vi "torres hanoi.vi"() -> ()   [LabVIEW 2020]
uses:
  <vilib>/Utility/miscctls.llb/LVPoint32TypeDef.ctl
  <vilib>/Utility/miscctls.llb/LVPositionTypeDef.ctl
  <vilib>/Utility/miscctls.llb/LVBoundsTypeDef.ctl
panel:
  out "?":string
  out "solucion de inicio a final 5":string
  out "solucion de inicio a final 4":string
  in  "?":bool
  out "solucion de inicio a final 3":string
  out "result":bool
  out "Position 1":T1
  out "# de movimientos":dbl
  out "Position 2":T1
  out "Position 3":T1
  out "Position 4":T1
  out "Position 5":T1
  out "Position":T1
  in  "seleccione  # de discos:":u16(ring) items=["3"=3, "4"=4, "5"=5]
  out "Coords":T2
  in  "?":bool
  out "disco5":bool
  out "disco4":bool
  out "disco3":bool
  out "disco2":bool
  out "disco1":bool
  out "final":bool
  out "medio":bool
  out "inicio":bool
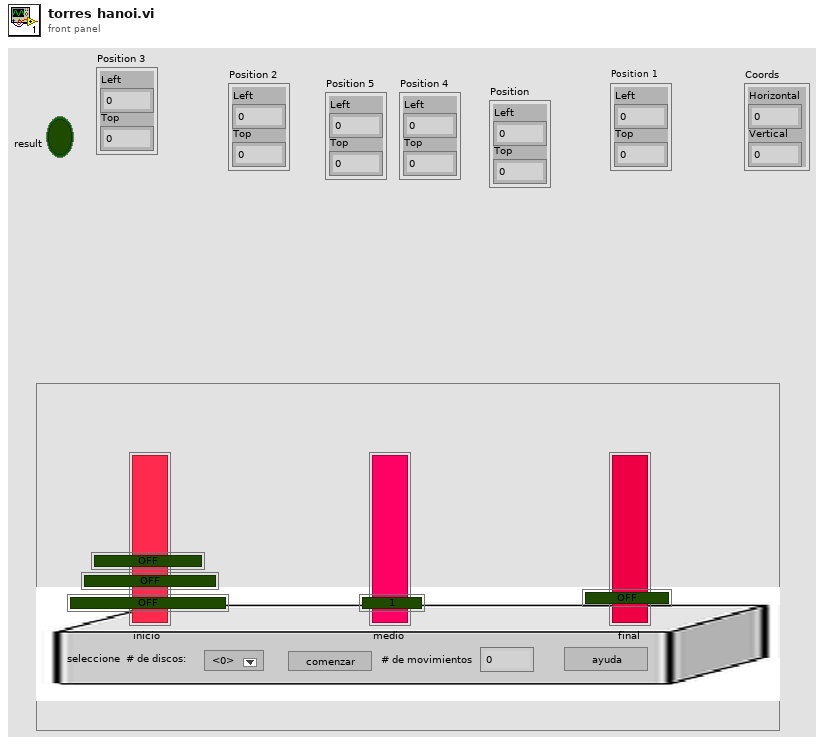
[diagram p1: front panel]
types:
  T1 = typedef "LVPositionTypeDef.ctl" = cluster{"Left":i32, "Top":i32}
  T2 = typedef "LVPoint32TypeDef.ctl" = cluster{"Horizontal":i32, "Vertical":i32}
  T3 = typedef "LVBoundsTypeDef.ctl" = cluster{"Width":u32, "Height":u32}
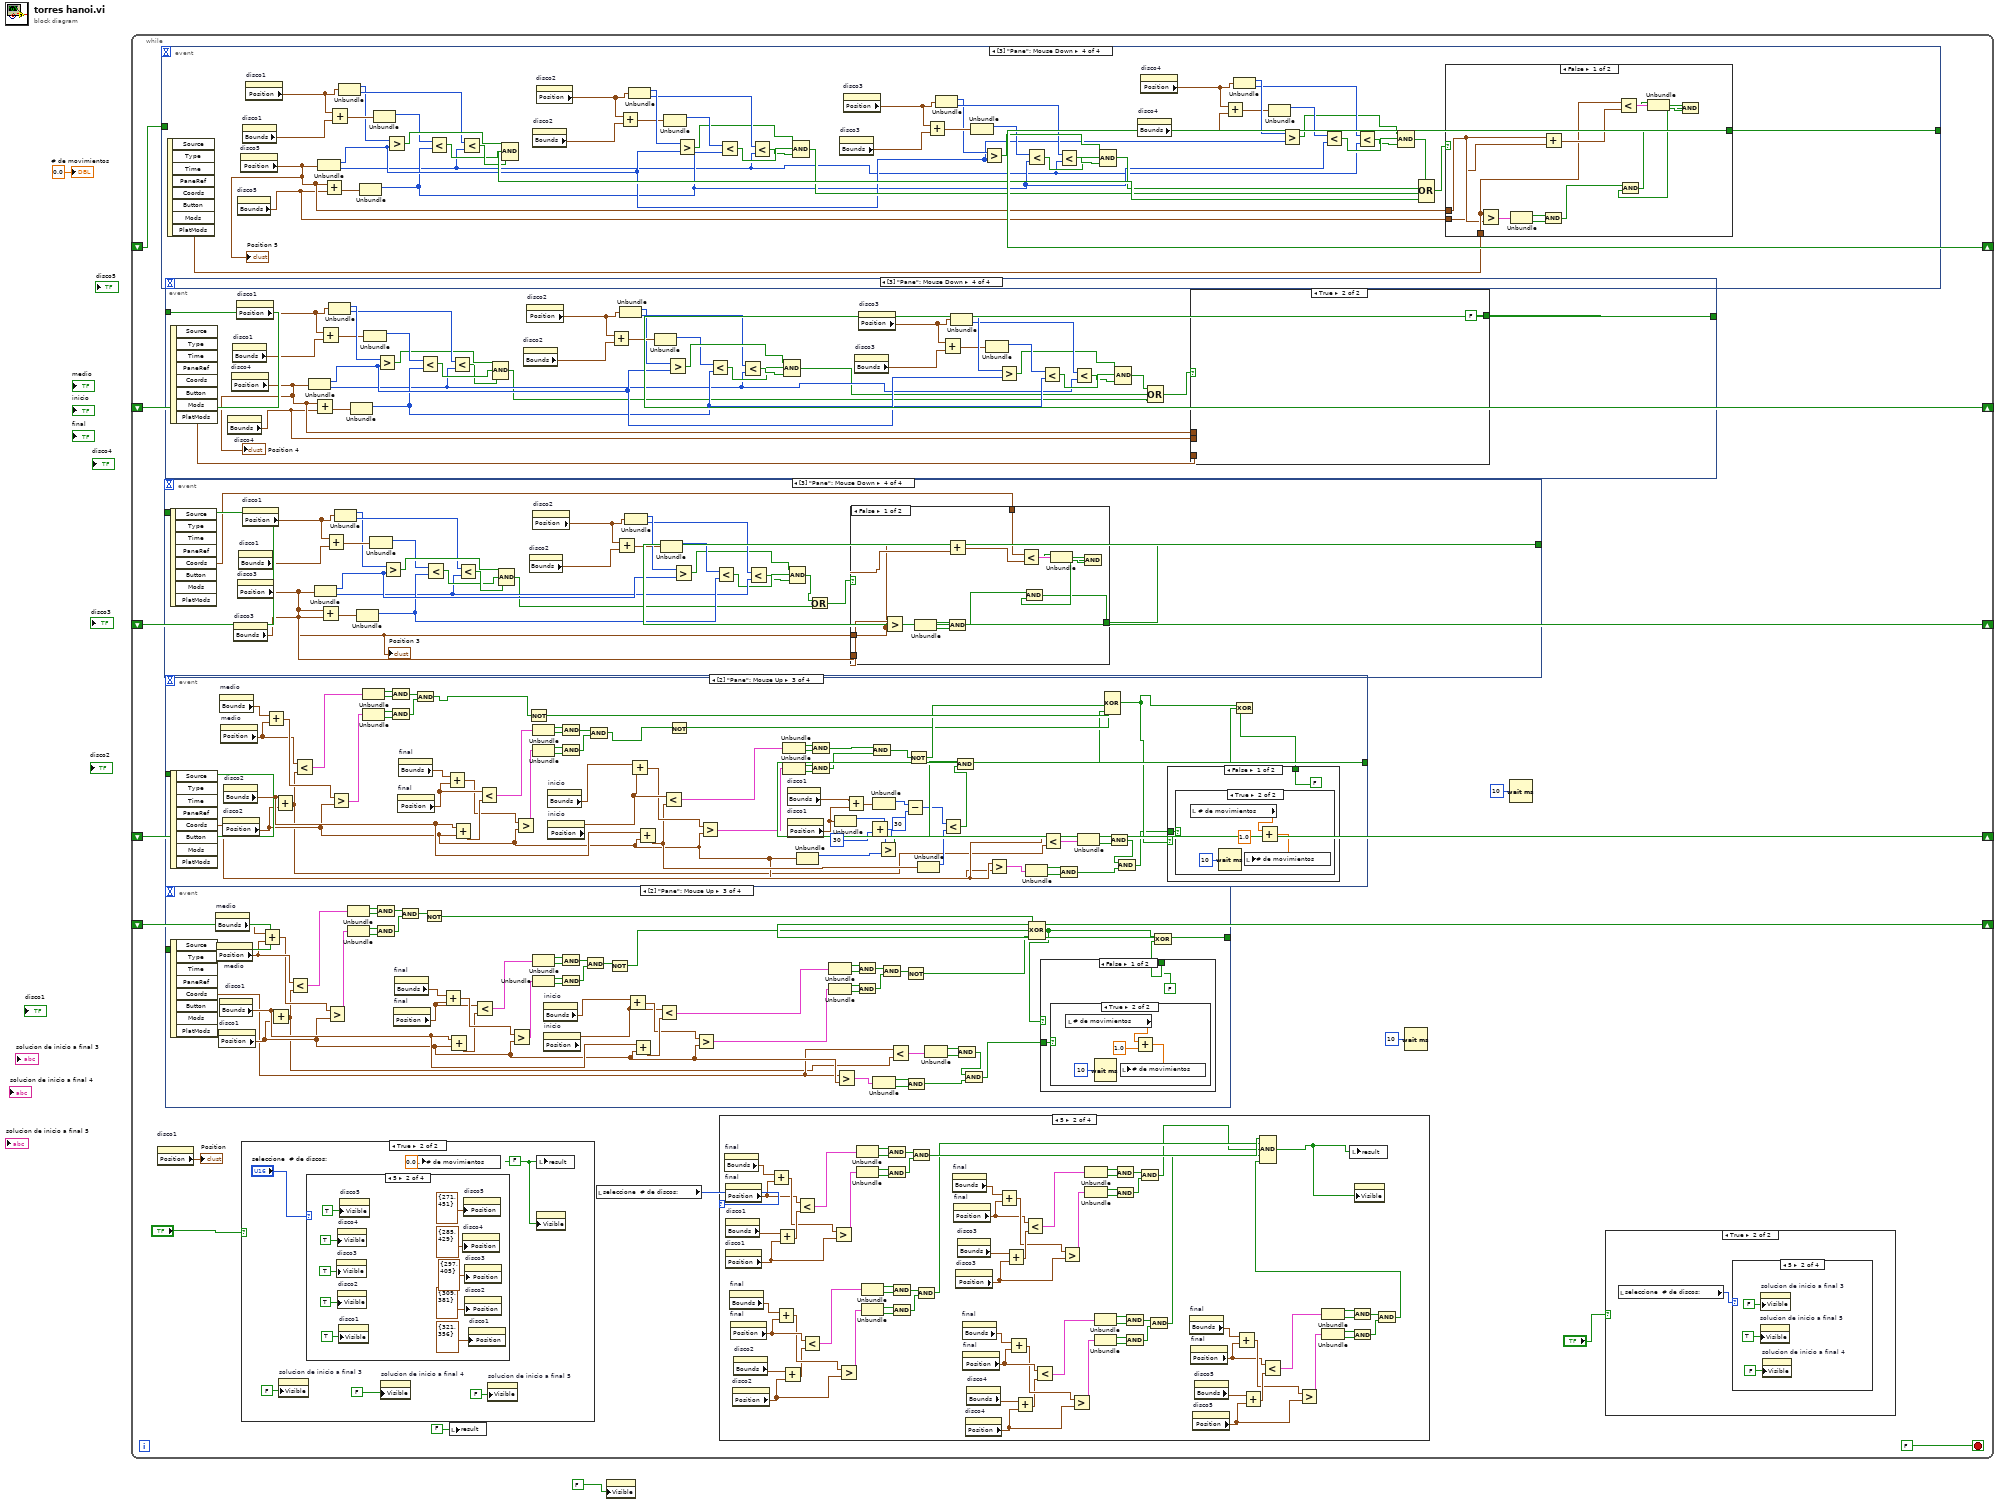
[diagram p0: block diagram]
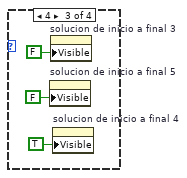
[diagram p4: hidden frame]
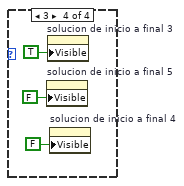
[diagram p5: hidden frame]
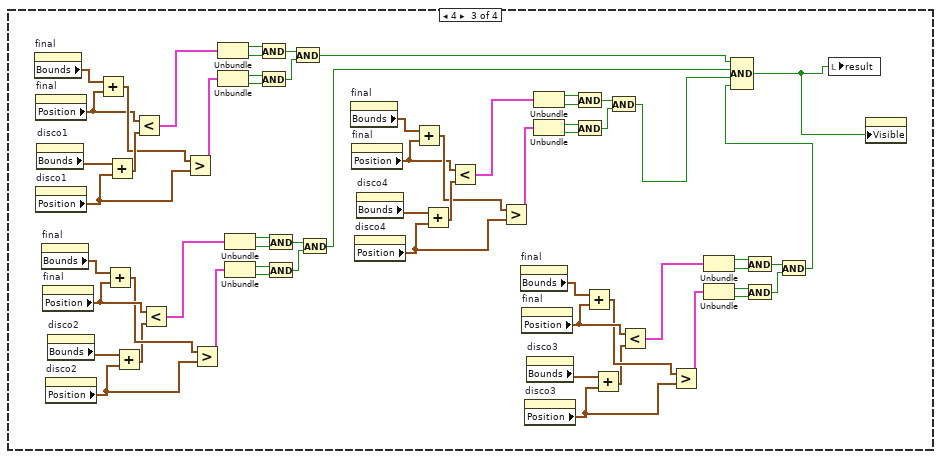
[diagram p7: hidden frame]
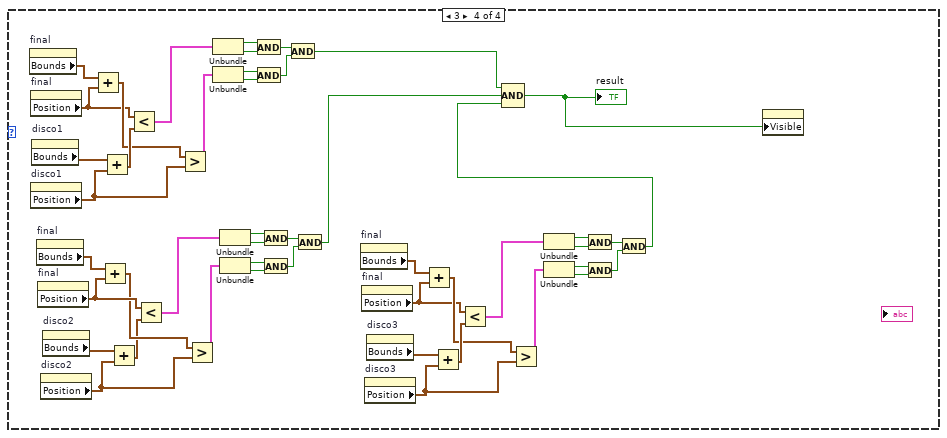
[diagram p8: hidden frame]
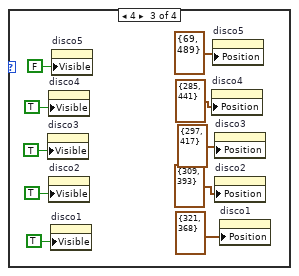
[diagram p11: hidden frame]
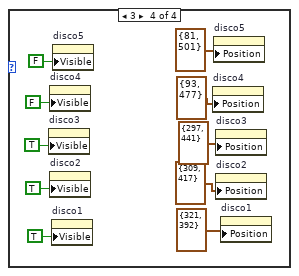
[diagram p12: hidden frame]
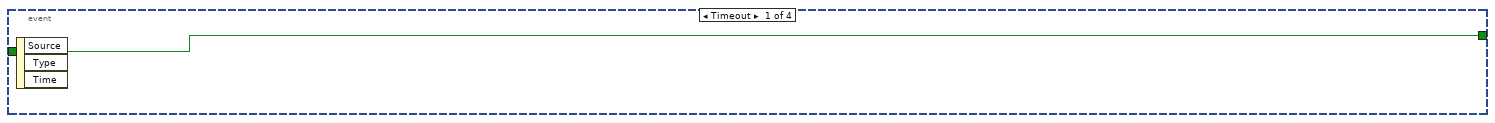
[diagram p13: hidden frame]
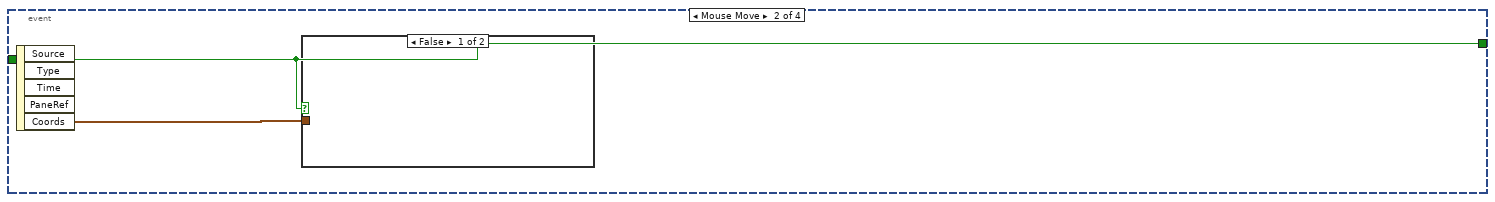
[diagram p14: hidden frame]
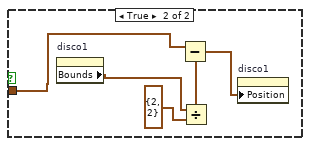
[diagram p15: hidden frame]
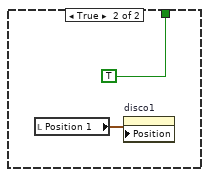
[diagram p17: hidden frame]
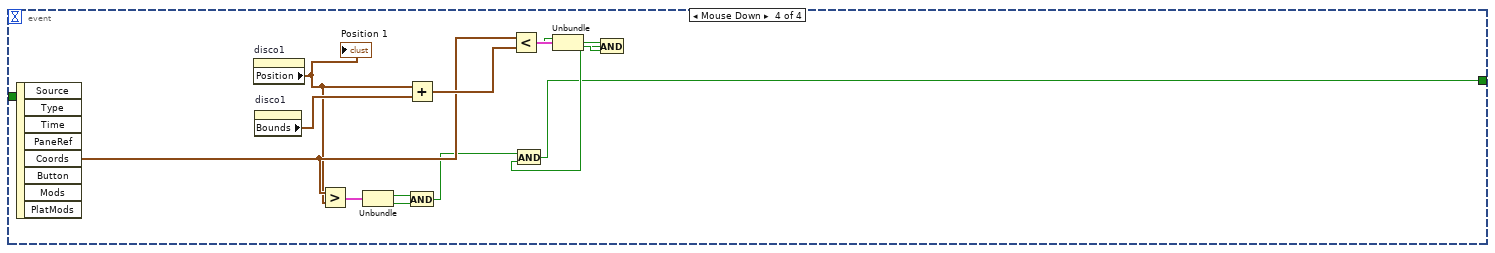
[diagram p18: hidden frame]
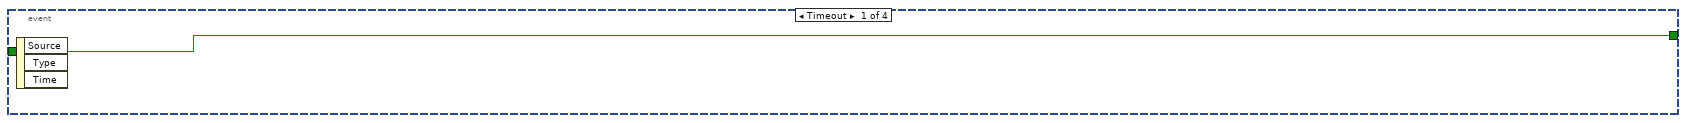
[diagram p19: hidden frame]
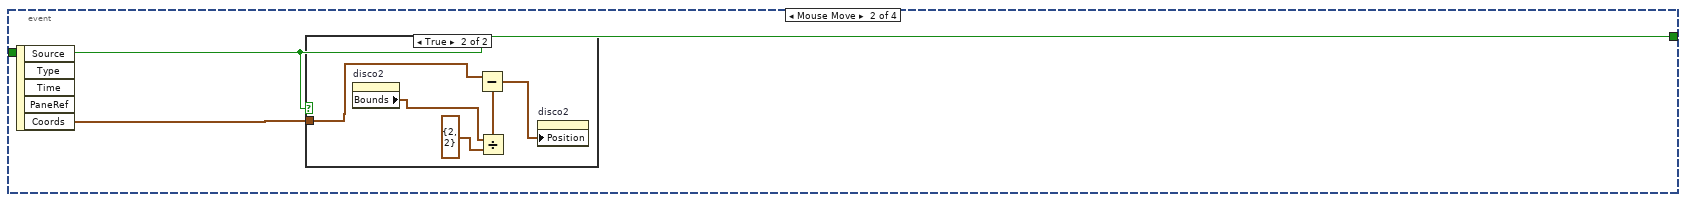
[diagram p20: hidden frame]
diagram:
  n1 = while {
    shift-right: [w18] -> _
    shift-left: _ -> [w19]
    shift-right: [w16] -> _
    shift-left: _ -> [w17]
    shift-right: [w14] -> _
    shift-left: _ -> [w15]
    shift-right: [w12] -> _
    shift-left: _ -> [w13]
    shift-right: [w10] -> _
    shift-left: _ -> [w11]
    stop <- FALSE stop-if-true
    n2 = property on="disco1" class="Bool (strict)"() -> ("Position"=→"Position":T1)  [unwired: 2 in, 2 out]
    n3 = event shown="[3] \"Pane\": Mouse Down" {
      selector: _ -> [_ _ _ _]
      dyn-events: _ -> [_ _ _ _]
      timeout: _ -> [_ _ _ _]
      tunnel: w19 -> [w764 w765 _ _]
      tunnel: [w764 w765 w836 w935] -> w18
      event Timeout {
        n4 = event-data() -> ()  [unwired: 1 in, 3 out]
      }
      event Mouse Move {
        n5 = event-data() -> ("Coords"=w766:T2)  [unwired: 1 in, 4 out]
        n6 = case shown="False" w765 {
          tunnel: w766 -> [_ w769]
          frame False {
          }
          frame True {
            n7 = property on="disco5" class="Bool (strict)"() -> ("Bounds"=w771:T3)  [unwired: 2 in, 2 out]
            n8 = Divide(x=w771, y=T3 {"Width"=2, "Height"=2}) -> (x/y=w768:cluster{"Width":dbl, "Height":dbl})
            n9 = Subtract(x=w769, y=w768) -> (x-y=w767:cluster{dbl, dbl})
            n10 = property on="disco5" class="Bool (strict)"("Position"=w767) -> ()  [unwired: 2 in, 2 out]
            "Coords" <- w769
          }
        }
      }
      event Mouse Up {
        n11 = event-data() -> ("Coords"=w774:T2)  [unwired: 1 in, 7 out]
        n12 = property on="medio" class="Bool (strict)"() -> ("Bounds"=w871:T3)  [unwired: 2 in, 2 out]
        n13 = property on="medio" class="Bool (strict)"() -> ("Position"=w870:T1)  [unwired: 2 in, 2 out]
        n14 = property on="disco5" class="Bool (strict)"() -> ("Position"=w773:T1)  [unwired: 2 in, 2 out]
        n15 = property on="disco5" class="Bool (strict)"() -> ("Bounds"=w842:T3)  [unwired: 2 in, 2 out]
        n16 = Add(x=w871, y=w870) -> (x+y=w869:T3)
        n17 = Add(x=w842, y=w773) -> (x+y=w772:T3)
        n18 = Less?(x=w870, y=w772) -> (x < y?=w873:cluster{bool, bool})
        n19 = Greater?(x=w869, y=w773) -> (0:w872:cluster{bool, bool})
        n20 = Unbundle(w873) -> (w877:bool, w876:bool)
        n21 = Unbundle(w872) -> (w879:bool, w878:bool)
        n22 = And(x=w877, y=w876) -> (x .and. y?=w874:bool)
        n23 = And(x=w879, y=w878) -> (x .and. y?=w875:bool)
        n24 = property on="final" class="Bool (strict)"() -> ("Position"=w855:T1)  [unwired: 2 in, 2 out]
        n25 = property on="final" class="Bool (strict)"() -> ("Bounds"=w856:T3)  [unwired: 2 in, 2 out]
        n26 = And(x=w874, y=w875) -> (x .and. y?=w868:bool)
        n27 = Not(x=w868) -> (.not. x?=w839:bool)
        n28 = Add(x=w856, y=w855) -> (x+y=w866:T3)
        n29 = Add(x=w842, y=w773) -> (x+y=w863:T3)
        n30 = Less?(x=w855, y=w863) -> (x < y?=w864:cluster{bool, bool})
        n31 = Greater?(x=w866, y=w773) -> (0:w865:cluster{bool, bool})
        n32 = Unbundle(w864) -> (w859:bool, w860:bool)
        n33 = Unbundle(w865) -> (w857:bool, w858:bool)
        n34 = property on="inicio" class="Bool (strict)"() -> ("Bounds"=w844:T3)  [unwired: 2 in, 2 out]
        n35 = property on="inicio" class="Bool (strict)"() -> ("Position"=w843:T1)  [unwired: 2 in, 2 out]
        n36 = And(x=w859, y=w860) -> (x .and. y?=w862:bool)
        n37 = And(x=w857, y=w858) -> (x .and. y?=w861:bool)
        n38 = And(x=w862, y=w861) -> (x .and. y?=w867:bool)
        n39 = Not(x=w867) -> (.not. x?=w840:bool)
        n40 = Add(x=w844, y=w843) -> (x+y=w846:T3)
        n41 = Add(x=w842, y=w773) -> (x+y=w824:T3)
        n42 = Less?(x=w843, y=w824) -> (x < y?=w848:cluster{bool, bool})
        n43 = Greater?(x=w846, y=w773) -> (0:w847:cluster{bool, bool})
        n44 = Unbundle(w848) -> (w852:bool, w851:bool)
        n45 = Unbundle(w847) -> (w854:bool, w853:bool)
        n46 = property on="disco1" class="Bool (strict)"() -> ("Bounds"=w830:T3)  [unwired: 2 in, 2 out]
        n47 = property on="disco1" class="Bool (strict)"() -> ("Position"=w831:T1)  [unwired: 2 in, 2 out]
        n48 = Unbundle(w773) -> ("Left"=w814:i32)  [unwired: 1 out]
        n49 = And(x=w852, y=w851) -> (x .and. y?=w849:bool)
        n50 = And(x=w854, y=w853) -> (x .and. y?=w850:bool)
        n51 = And(x=w849, y=w850) -> (x .and. y?=w845:bool)
        n52 = Unbundle(w831) -> ("Left"=w812:i32)  [unwired: 1 out]
        n53 = Add(x=w830, y=w831) -> (x+y=w832:T3)
        n54 = Not(x=w845) -> (.not. x?=w841:bool)
        n55 = Add(x=w812, y=30) -> (x+y=w810:i32)
        n56 = Greater?(x=w810, y=w814) -> (0:w826:bool)
        n57 = Unbundle(w832) -> ("Width"=w809:u32)  [unwired: 1 out]
        n58 = Subtract(x=w809, y=u32 30) -> (x-y=w807:u32)
        n59 = Unbundle(w824) -> ("Width"=w813:u32)  [unwired: 1 out]
        n60 = Less?(x=w807, y=w813) -> (x < y?=w825:bool)
        n61 = And(x=w826, y=w825) -> (x .and. y?=w784:bool)
        n62 = property on="disco2" class="Bool (strict)"() -> ("Bounds"=w829:T3)  [unwired: 2 in, 2 out]
        n63 = property on="disco2" class="Bool (strict)"() -> ("Position"=w828:T1)  [unwired: 2 in, 2 out]
        n64 = Unbundle(w828) -> ("Left"=w805:i32)  [unwired: 1 out]
        n65 = Add(x=w829, y=w828) -> (x+y=w827:T3)
        n66 = Add(x=w805, y=30) -> (x+y=w806:i32)
        n67 = Unbundle(w827) -> ("Width"=w803:u32)  [unwired: 1 out]
        n68 = Greater?(x=w806, y=w814) -> (0:w823:bool)
        n69 = Subtract(x=w803, y=u32 30) -> (x-y=w802:u32)
        n70 = Less?(x=w802, y=w813) -> (x < y?=w822:bool)
        n71 = And(x=w823, y=w822) -> (x .and. y?=w785:bool)
        n72 = property on="disco3" class="Bool (strict)"() -> ("Bounds"=w833:T3)  [unwired: 2 in, 2 out]
        n73 = property on="disco3" class="Bool (strict)"() -> ("Position"=w834:T1)  [unwired: 2 in, 2 out]
        n74 = Unbundle(w834) -> ("Left"=w800:i32)  [unwired: 1 out]
        n75 = Add(x=w833, y=w834) -> (x+y=w835:T3)
        n76 = Add(x=w800, y=30) -> (x+y=w799:i32)
        n77 = Unbundle(w835) -> ("Width"=w797:u32)  [unwired: 1 out]
        n78 = Greater?(x=w799, y=w814) -> (0:w821:bool)
        n79 = Subtract(x=w797, y=u32 30) -> (x-y=w796:u32)
        n80 = Less?(x=w796, y=w813) -> (x < y?=w820:bool)
        n81 = And(x=w821, y=w820) -> (x .and. y?=w786:bool)
        n82 = property on="disco4" class="Bool (strict)"() -> ("Bounds"=w817:T3)  [unwired: 2 in, 2 out]
        n83 = property on="disco4" class="Bool (strict)"() -> ("Position"=w816:T1)  [unwired: 2 in, 2 out]
        n84 = Unbundle(w816) -> ("Left"=w794:i32)  [unwired: 1 out]
        n85 = Add(x=w817, y=w816) -> (x+y=w815:T3)
        n86 = Add(x=w794, y=30) -> (x+y=w793:i32)
        n87 = Greater?(x=w793, y=w814) -> (0:w818:bool)
        n88 = Unbundle(w815) -> ("Width"=w791:u32)  [unwired: 1 out]
        n89 = Subtract(x=w791, y=u32 30) -> (x-y=w789:u32)
        n90 = Less?(x=w789, y=w813) -> (x < y?=w819:bool)
        n91 = And(x=w818, y=w819) -> (x .and. y?=w787:bool)
        n92 = Compound Arithmetic op=OR(w784, w785, w786, w787) -> (w788:bool)
        n93 = Greater?(x=w774, y=w773) -> (0:w783:cluster{bool, bool})
        n94 = Unbundle(w783) -> (w781:bool, w780:bool)
        n95 = Less?(x=w774, y=w772) -> (x < y?=w782:cluster{bool, bool})
        n96 = And(x=w781, y=w780) -> (x .and. y?=w776:bool)
        n97 = Unbundle(w782) -> (w779:bool, w778:bool)
        n98 = And(x=w779, y=w778) -> (x .and. y?=w777:bool)
        n99 = And(x=w777, y=w776) -> (x .and. y?=w775:bool)
        n100 = Compound Arithmetic op=XOR(w839, w840, w841, w788) -> (w837:bool)
        n101 = case shown="False" w837 {
          tunnel: [FALSE ("Accepted?") TRUE ("Accepted?")] -> w838
          tunnel: w775 -> [w880 _]
          frame False {
            n102 = case shown="True" w880 {
              frame False {
              }
              frame True {
                n103 = local read "# de movimientos"() -> (w884:dbl)
                n104 = Wait (ms)(milliseconds to wait=u32 10) -> ()  [unwired: 1 out]
                n105 = Add(x=w884, y=1.0) -> (x+y=w885:dbl)
                n106 = local write "# de movimientos"(w885) -> ()
              }
            }
          }
          frame True {
            n107 = local read "Position 5"() -> (w887:T1)
            n108 = property on="disco5" class="Bool (strict)"("Position"=w887) -> ()  [unwired: 2 in, 2 out]
          }
        }
        n109 = Exclusive Or(1:w838, 2:w837) -> (0:w836:bool)
      }
      event Mouse Down {
        n110 = event-data() -> ("Coords"=w936:T2)  [unwired: 1 in, 7 out]
        n111 = property on="disco5" class="Bool (strict)"() -> ("Bounds"=w902:T3)  [unwired: 2 in, 2 out]
        n112 = property on="disco5" class="Bool (strict)"() -> ("Position"=w903:T1)  [unwired: 2 in, 2 out]
        "Position 5" <- w903
        n113 = property on="disco1" class="Bool (strict)"() -> ("Bounds"=w913:T3)  [unwired: 2 in, 2 out]
        n114 = property on="disco1" class="Bool (strict)"() -> ("Position"=w914:T1)  [unwired: 2 in, 2 out]
        n115 = Unbundle(w903) -> ("Left"=w891:i32, "Top"=w889:i32)
        n116 = Add(x=w903, y=w902) -> (x+y=w917:T3)
        n117 = Add(x=w914, y=w913) -> (x+y=w916:T3)
        n118 = Unbundle(w914) -> ("Left"=w915:i32, "Top"=w919:i32)
        n119 = Unbundle(w917) -> ("Width"=w890:u32)  [unwired: 1 out]
        n120 = Unbundle(w916) -> ("Width"=w918:u32)  [unwired: 1 out]
        n121 = Greater?(x=w915, y=w891) -> (0:w920:bool)
        n122 = Less?(x=w918, y=w890) -> (x < y?=w921:bool)
        n123 = Less?(x=w919, y=w889) -> (x < y?=w922:bool)
        n124 = Compound Arithmetic op=AND(w920, w921, w922) -> (w934:bool)
        n125 = property on="disco2" class="Bool (strict)"() -> ("Bounds"=w912:T3)  [unwired: 2 in, 2 out]
        n126 = property on="disco2" class="Bool (strict)"() -> ("Position"=w911:T1)  [unwired: 2 in, 2 out]
        n127 = Add(x=w911, y=w912) -> (x+y=w909:T3)
        n128 = Unbundle(w911) -> ("Left"=w910:i32, "Top"=w907:i32)
        n129 = Unbundle(w909) -> ("Width"=w908:u32)  [unwired: 1 out]
        n130 = Greater?(x=w910, y=w891) -> (0:w906:bool)
        n131 = Less?(x=w908, y=w890) -> (x < y?=w905:bool)
        n132 = Less?(x=w907, y=w889) -> (x < y?=w904:bool)
        n133 = Compound Arithmetic op=AND(w906, w905, w904) -> (w933:bool)
        n134 = property on="disco3" class="Bool (strict)"() -> ("Bounds"=w923:T3)  [unwired: 2 in, 2 out]
        n135 = property on="disco3" class="Bool (strict)"() -> ("Position"=w924:T1)  [unwired: 2 in, 2 out]
        n136 = Add(x=w924, y=w923) -> (x+y=w926:T3)
        n137 = Unbundle(w924) -> ("Left"=w925:i32, "Top"=w928:i32)
        n138 = Unbundle(w926) -> ("Width"=w927:u32)  [unwired: 1 out]
        n139 = Greater?(x=w925, y=w891) -> (0:w929:bool)
        n140 = Less?(x=w927, y=w890) -> (x < y?=w930:bool)
        n141 = Less?(x=w928, y=w889) -> (x < y?=w931:bool)
        n142 = Compound Arithmetic op=AND(w929, w930, w931) -> (w932:bool)
        n143 = property on="disco4" class="Bool (strict)"() -> ("Bounds"=w901:T3)  [unwired: 2 in, 2 out]
        n144 = property on="disco4" class="Bool (strict)"() -> ("Position"=w900:T1)  [unwired: 2 in, 2 out]
        n145 = Add(x=w900, y=w901) -> (x+y=w898:T3)
        n146 = Unbundle(w900) -> ("Left"=w899:i32, "Top"=w896:i32)
        n147 = Unbundle(w898) -> ("Width"=w897:u32)  [unwired: 1 out]
        n148 = Greater?(x=w899, y=w891) -> (0:w895:bool)
        n149 = Less?(x=w897, y=w890) -> (x < y?=w894:bool)
        n150 = Less?(x=w896, y=w889) -> (x < y?=w893:bool)
        n151 = Compound Arithmetic op=AND(w895, w894, w893) -> (w892:bool)
        n152 = Compound Arithmetic op=OR(w892, w932, w933, w934) -> (w888:bool)
        n153 = case shown="False" w888 {
          tunnel: w936 -> [w948 _]
          tunnel: [w939 FALSE] -> w935
          tunnel: w903 -> [w938 _]
          tunnel: w902 -> [w937 _]
          frame False {
            n154 = Greater?(x=w948, y=w938) -> (0:w947:cluster{bool, bool})
            n155 = Unbundle(w947) -> (w943:bool, w942:bool)
            n156 = Add(x=w938, y=w937) -> (x+y=w949:T3)
            n157 = And(x=w943, y=w942) -> (x .and. y?=w940:bool)
            n158 = Less?(x=w948, y=w949) -> (x < y?=w946:cluster{bool, bool})
            n159 = Unbundle(w946) -> (w945:bool, w944:bool)
            n160 = And(x=w945, y=w944) -> (x .and. y?=w941:bool)
            n161 = And(x=w940, y=w941) -> (x .and. y?=w939:bool)
          }
          frame True {
          }
        }
      }
    }
    n162 = event shown="[3] \"Pane\": Mouse Down" {
      selector: _ -> [_ _ _ _]
      dyn-events: _ -> [_ _ _ _]
      timeout: _ -> [_ _ _ _]
      tunnel: w15 -> [w456 w457 _ _]
      tunnel: [w456 w457 w504 w583] -> w14
      event Timeout {
        n163 = event-data() -> ()  [unwired: 1 in, 3 out]
      }
      event Mouse Move {
        n164 = event-data() -> ("Coords"=w458:T2)  [unwired: 1 in, 4 out]
        n165 = case shown="False" w457 {
          tunnel: w458 -> [_ w462]
          frame False {
          }
          frame True {
            n166 = property on="disco3" class="Bool (strict)"() -> ("Bounds"=w460:T3)  [unwired: 2 in, 2 out]
            n167 = Divide(x=w460, y=T3 {"Width"=2, "Height"=2}) -> (x/y=w461:cluster{"Width":dbl, "Height":dbl})
            n168 = Subtract(x=w462, y=w461) -> (x-y=w459:cluster{dbl, dbl})
            n169 = property on="disco3" class="Bool (strict)"("Position"=w459) -> ()  [unwired: 2 in, 2 out]
          }
        }
      }
      event Mouse Up {
        n170 = event-data() -> ("Coords"=w466:T2)  [unwired: 1 in, 7 out]
        n171 = property on="medio" class="Bool (strict)"() -> ("Bounds"=w539:T3)  [unwired: 2 in, 2 out]
        n172 = property on="medio" class="Bool (strict)"() -> ("Position"=w538:T1)  [unwired: 2 in, 2 out]
        n173 = property on="disco3" class="Bool (strict)"() -> ("Position"=w465:T1)  [unwired: 2 in, 2 out]
        n174 = property on="disco3" class="Bool (strict)"() -> ("Bounds"=w510:T3)  [unwired: 2 in, 2 out]
        n175 = Add(x=w539, y=w538) -> (x+y=w537:T3)
        n176 = Add(x=w510, y=w465) -> (x+y=w464:T3)
        n177 = Less?(x=w538, y=w464) -> (x < y?=w541:cluster{bool, bool})
        n178 = Greater?(x=w537, y=w465) -> (0:w540:cluster{bool, bool})
        n179 = Unbundle(w541) -> (w545:bool, w544:bool)
        n180 = Unbundle(w540) -> (w547:bool, w546:bool)
        n181 = And(x=w545, y=w544) -> (x .and. y?=w542:bool)
        n182 = And(x=w547, y=w546) -> (x .and. y?=w543:bool)
        n183 = property on="final" class="Bool (strict)"() -> ("Position"=w523:T1)  [unwired: 2 in, 2 out]
        n184 = property on="final" class="Bool (strict)"() -> ("Bounds"=w524:T3)  [unwired: 2 in, 2 out]
        n185 = And(x=w542, y=w543) -> (x .and. y?=w536:bool)
        n186 = Not(x=w536) -> (.not. x?=w507:bool)
        n187 = Add(x=w524, y=w523) -> (x+y=w534:T3)
        n188 = Add(x=w510, y=w465) -> (x+y=w531:T3)
        n189 = Less?(x=w523, y=w531) -> (x < y?=w532:cluster{bool, bool})
        n190 = Greater?(x=w534, y=w465) -> (0:w533:cluster{bool, bool})
        n191 = Unbundle(w532) -> (w527:bool, w528:bool)
        n192 = Unbundle(w533) -> (w525:bool, w526:bool)
        n193 = property on="inicio" class="Bool (strict)"() -> ("Bounds"=w512:T3)  [unwired: 2 in, 2 out]
        n194 = property on="inicio" class="Bool (strict)"() -> ("Position"=w511:T1)  [unwired: 2 in, 2 out]
        n195 = And(x=w527, y=w528) -> (x .and. y?=w530:bool)
        n196 = And(x=w525, y=w526) -> (x .and. y?=w529:bool)
        n197 = And(x=w530, y=w529) -> (x .and. y?=w535:bool)
        n198 = Not(x=w535) -> (.not. x?=w508:bool)
        n199 = Add(x=w512, y=w511) -> (x+y=w514:T3)
        n200 = Add(x=w510, y=w465) -> (x+y=w500:T3)
        n201 = Less?(x=w511, y=w500) -> (x < y?=w516:cluster{bool, bool})
        n202 = Greater?(x=w514, y=w465) -> (0:w515:cluster{bool, bool})
        n203 = Unbundle(w516) -> (w520:bool, w519:bool)
        n204 = Unbundle(w515) -> (w522:bool, w521:bool)
        n205 = And(x=w520, y=w519) -> (x .and. y?=w517:bool)
        n206 = And(x=w522, y=w521) -> (x .and. y?=w518:bool)
        n207 = And(x=w517, y=w518) -> (x .and. y?=w513:bool)
        n208 = property on="disco1" class="Bool (strict)"() -> ("Bounds"=w501:T3)  [unwired: 2 in, 2 out]
        n209 = property on="disco1" class="Bool (strict)"() -> ("Position"=w502:T1)  [unwired: 2 in, 2 out]
        n210 = Unbundle(w465) -> ("Left"=w494:i32)  [unwired: 1 out]
        n211 = Not(x=w513) -> (.not. x?=w509:bool)
        n212 = Unbundle(w502) -> ("Left"=w490:i32)  [unwired: 1 out]
        n213 = Add(x=w501, y=w502) -> (x+y=w503:T3)
        n214 = Add(x=w490, y=30) -> (x+y=w489:i32)
        n215 = Unbundle(w503) -> ("Width"=w486:u32)  [unwired: 1 out]
        n216 = Greater?(x=w489, y=w494) -> (0:w499:bool)
        n217 = Subtract(x=w486, y=u32 30) -> (x-y=w487:u32)
        n218 = Unbundle(w500) -> ("Width"=w493:u32)  [unwired: 1 out]
        n219 = Less?(x=w487, y=w493) -> (x < y?=w498:bool)
        n220 = And(x=w499, y=w498) -> (x .and. y?=w477:bool)
        n221 = property on="disco2" class="Bool (strict)"() -> ("Bounds"=w497:T3)  [unwired: 2 in, 2 out]
        n222 = property on="disco2" class="Bool (strict)"() -> ("Position"=w496:T1)  [unwired: 2 in, 2 out]
        n223 = Unbundle(w496) -> ("Left"=w484:i32)  [unwired: 1 out]
        n224 = Add(x=w497, y=w496) -> (x+y=w495:T3)
        n225 = Add(x=w484, y=30) -> (x+y=w483:i32)
        n226 = Unbundle(w495) -> ("Width"=w481:u32)  [unwired: 1 out]
        n227 = Greater?(x=w483, y=w494) -> (0:w491:bool)
        n228 = Subtract(x=w481, y=u32 30) -> (x-y=w480:u32)
        n229 = Less?(x=w480, y=w493) -> (x < y?=w492:bool)
        n230 = And(x=w491, y=w492) -> (x .and. y?=w478:bool)
        n231 = Or(x=w477, y=w478) -> (x .or. y?=w476:bool)
        n232 = Greater?(x=w466, y=w465) -> (0:w475:cluster{bool, bool})
        n233 = Unbundle(w475) -> (w473:bool, w472:bool)
        n234 = Less?(x=w466, y=w464) -> (x < y?=w474:cluster{bool, bool})
        n235 = And(x=w473, y=w472) -> (x .and. y?=w468:bool)
        n236 = Unbundle(w474) -> (w471:bool, w470:bool)
        n237 = And(x=w471, y=w470) -> (x .and. y?=w469:bool)
        n238 = And(x=w469, y=w468) -> (x .and. y?=w467:bool)
        n239 = Compound Arithmetic op=XOR(w507, w508, w509, w476) -> (w505:bool)
        n240 = case shown="False" w505 {
          tunnel: [FALSE ("Accepted?") TRUE ("Accepted?")] -> w506
          tunnel: w467 -> [w548 _]
          frame False {
            n241 = case shown="True" w548 {
              frame False {
              }
              frame True {
                n242 = local read "# de movimientos"() -> (w552:dbl)
                n243 = Wait (ms)(milliseconds to wait=u32 10) -> ()  [unwired: 1 out]
                n244 = Add(x=w552, y=1.0) -> (x+y=w553:dbl)
                n245 = local write "# de movimientos"(w553) -> ()
              }
            }
          }
          frame True {
            n246 = local read "Position 3"() -> (w555:T1)
            n247 = property on="disco3" class="Bool (strict)"("Position"=w555) -> ()  [unwired: 2 in, 2 out]
          }
        }
        n248 = Exclusive Or(1:w506, 2:w505) -> (0:w504:bool)
      }
      event Mouse Down {
        n249 = event-data() -> ("Coords"=w584:T2)  [unwired: 1 in, 7 out]
        n250 = property on="disco3" class="Bool (strict)"() -> ("Bounds"=w572:T3)  [unwired: 2 in, 2 out]
        n251 = property on="disco3" class="Bool (strict)"() -> ("Position"=w571:T1)  [unwired: 2 in, 2 out]
        "Position 3" <- w571
        n252 = property on="disco1" class="Bool (strict)"() -> ("Bounds"=w573:T3)  [unwired: 2 in, 2 out]
        n253 = property on="disco1" class="Bool (strict)"() -> ("Position"=w574:T1)  [unwired: 2 in, 2 out]
        n254 = Unbundle(w571) -> ("Left"=w563:i32, "Top"=w561:i32)
        n255 = Add(x=w571, y=w572) -> (x+y=w577:T3)
        n256 = Add(x=w574, y=w573) -> (x+y=w576:T3)
        n257 = Unbundle(w574) -> ("Left"=w575:i32, "Top"=w579:i32)
        n258 = Unbundle(w577) -> ("Width"=w562:u32)  [unwired: 1 out]
        n259 = Unbundle(w576) -> ("Width"=w578:u32)  [unwired: 1 out]
        n260 = Greater?(x=w575, y=w563) -> (0:w580:bool)
        n261 = Less?(x=w578, y=w562) -> (x < y?=w581:bool)
        n262 = Less?(x=w579, y=w561) -> (x < y?=w582:bool)
        n263 = Compound Arithmetic op=AND(w580, w581, w582) -> (w556:bool)
        n264 = property on="disco2" class="Bool (strict)"() -> ("Bounds"=w570:T3)  [unwired: 2 in, 2 out]
        n265 = property on="disco2" class="Bool (strict)"() -> ("Position"=w569:T1)  [unwired: 2 in, 2 out]
        n266 = Add(x=w569, y=w570) -> (x+y=w567:T3)
        n267 = Unbundle(w569) -> ("Left"=w568:i32, "Top"=w565:i32)
        n268 = Unbundle(w567) -> ("Width"=w566:u32)  [unwired: 1 out]
        n269 = Greater?(x=w568, y=w563) -> (0:w564:bool)
        n270 = Less?(x=w566, y=w562) -> (x < y?=w560:bool)
        n271 = Less?(x=w565, y=w561) -> (x < y?=w559:bool)
        n272 = Compound Arithmetic op=AND(w564, w560, w559) -> (w557:bool)
        n273 = Or(x=w557, y=w556) -> (x .or. y?=w558:bool)
        n274 = case shown="False" w558 {
          tunnel: w584 -> [w588 _]
          tunnel: [w587 FALSE] -> w583
          tunnel: w572 -> [w586 _]
          tunnel: w571 -> [w585 _]
          frame False {
            n275 = Greater?(x=w588, y=w585) -> (0:w596:cluster{bool, bool})
            n276 = Unbundle(w596) -> (w592:bool, w591:bool)
            n277 = Add(x=w585, y=w586) -> (x+y=w597:T3)
            n278 = And(x=w592, y=w591) -> (x .and. y?=w589:bool)
            n279 = Less?(x=w588, y=w597) -> (x < y?=w595:cluster{bool, bool})
            n280 = Unbundle(w595) -> (w594:bool, w593:bool)
            n281 = And(x=w594, y=w593) -> (x .and. y?=w590:bool)
            n282 = And(x=w589, y=w590) -> (x .and. y?=w587:bool)
          }
          frame True {
          }
        }
      }
    }
    n283 = event shown="[3] \"Pane\": Mouse Down" {
      selector: _ -> [_ _ _ _]
      dyn-events: _ -> [_ _ _ _]
      timeout: _ -> [_ _ _ _]
      tunnel: w17 -> [w599 w600 _ _]
      tunnel: [w599 w600 w660 w748] -> w16
      event Timeout {
        n284 = event-data() -> ()  [unwired: 1 in, 3 out]
      }
      event Mouse Move {
        n285 = event-data() -> ("Coords"=w601:T2)  [unwired: 1 in, 4 out]
        n286 = case shown="False" w600 {
          tunnel: w601 -> [_ w602]
          frame False {
          }
          frame True {
            n287 = property on="disco4" class="Bool (strict)"() -> ("Bounds"=w604:T3)  [unwired: 2 in, 2 out]
            n288 = Divide(x=w604, y=T3 {"Width"=2, "Height"=2}) -> (x/y=w605:cluster{"Width":dbl, "Height":dbl})
            n289 = Subtract(x=w602, y=w605) -> (x-y=w603:cluster{dbl, dbl})
            n290 = property on="disco4" class="Bool (strict)"("Position"=w603) -> ()  [unwired: 2 in, 2 out]
          }
        }
      }
      event Mouse Up {
        n291 = event-data() -> ("Coords"=w609:T2)  [unwired: 1 in, 7 out]
        n292 = property on="medio" class="Bool (strict)"() -> ("Bounds"=w669:T3)  [unwired: 2 in, 2 out]
        n293 = property on="medio" class="Bool (strict)"() -> ("Position"=w670:T1)  [unwired: 2 in, 2 out]
        n294 = property on="disco4" class="Bool (strict)"() -> ("Position"=w608:T1)  [unwired: 2 in, 2 out]
        n295 = property on="disco4" class="Bool (strict)"() -> ("Bounds"=w698:T3)  [unwired: 2 in, 2 out]
        n296 = Add(x=w669, y=w670) -> (x+y=w671:T3)
        n297 = Add(x=w698, y=w608) -> (x+y=w607:T3)
        n298 = Less?(x=w670, y=w607) -> (x < y?=w667:cluster{bool, bool})
        n299 = Greater?(x=w671, y=w608) -> (0:w668:cluster{bool, bool})
        n300 = Unbundle(w667) -> (w663:bool, w664:bool)
        n301 = Unbundle(w668) -> (w661:bool, w662:bool)
        n302 = And(x=w663, y=w664) -> (x .and. y?=w666:bool)
        n303 = And(x=w661, y=w662) -> (x .and. y?=w665:bool)
        n304 = property on="final" class="Bool (strict)"() -> ("Position"=w685:T1)  [unwired: 2 in, 2 out]
        n305 = property on="final" class="Bool (strict)"() -> ("Bounds"=w684:T3)  [unwired: 2 in, 2 out]
        n306 = And(x=w666, y=w665) -> (x .and. y?=w672:bool)
        n307 = Not(x=w672) -> (.not. x?=w700:bool)
        n308 = Add(x=w684, y=w685) -> (x+y=w674:T3)
        n309 = Add(x=w698, y=w608) -> (x+y=w677:T3)
        n310 = Less?(x=w685, y=w677) -> (x < y?=w676:cluster{bool, bool})
        n311 = Greater?(x=w674, y=w608) -> (0:w675:cluster{bool, bool})
        n312 = Unbundle(w676) -> (w681:bool, w680:bool)
        n313 = Unbundle(w675) -> (w683:bool, w682:bool)
        n314 = property on="inicio" class="Bool (strict)"() -> ("Bounds"=w696:T3)  [unwired: 2 in, 2 out]
        n315 = property on="inicio" class="Bool (strict)"() -> ("Position"=w697:T1)  [unwired: 2 in, 2 out]
        n316 = And(x=w681, y=w680) -> (x .and. y?=w678:bool)
        n317 = And(x=w683, y=w682) -> (x .and. y?=w679:bool)
        n318 = And(x=w678, y=w679) -> (x .and. y?=w673:bool)
        n319 = Not(x=w673) -> (.not. x?=w699:bool)
        n320 = Add(x=w696, y=w697) -> (x+y=w694:T3)
        n321 = Add(x=w698, y=w608) -> (x+y=w649:T3)
        n322 = Less?(x=w697, y=w649) -> (x < y?=w692:cluster{bool, bool})
        n323 = Greater?(x=w694, y=w608) -> (0:w693:cluster{bool, bool})
        n324 = Unbundle(w692) -> (w688:bool, w689:bool)
        n325 = Unbundle(w693) -> (w686:bool, w687:bool)
        n326 = And(x=w688, y=w689) -> (x .and. y?=w691:bool)
        n327 = And(x=w686, y=w687) -> (x .and. y?=w690:bool)
        n328 = And(x=w691, y=w690) -> (x .and. y?=w695:bool)
        n329 = property on="disco1" class="Bool (strict)"() -> ("Bounds"=w656:T3)  [unwired: 2 in, 2 out]
        n330 = property on="disco1" class="Bool (strict)"() -> ("Position"=w655:T1)  [unwired: 2 in, 2 out]
        n331 = Unbundle(w608) -> ("Left"=w645:i32)  [unwired: 1 out]
        n332 = Not(x=w695) -> (.not. x?=w620:bool)
        n333 = Unbundle(w655) -> ("Left"=w641:i32)  [unwired: 1 out]
        n334 = Add(x=w656, y=w655) -> (x+y=w654:T3)
        n335 = Add(x=w641, y=30) -> (x+y=w639:i32)
        n336 = Unbundle(w654) -> ("Width"=w638:u32)  [unwired: 1 out]
        n337 = Greater?(x=w639, y=w645) -> (0:w651:bool)
        n338 = Subtract(x=w638, y=u32 30) -> (x-y=w637:u32)
        n339 = Unbundle(w649) -> ("Width"=w644:u32)  [unwired: 1 out]
        n340 = Less?(x=w637, y=w644) -> (x < y?=w650:bool)
        n341 = And(x=w651, y=w650) -> (x .and. y?=w621:bool)
        n342 = property on="disco2" class="Bool (strict)"() -> ("Bounds"=w657:T3)  [unwired: 2 in, 2 out]
        n343 = property on="disco2" class="Bool (strict)"() -> ("Position"=w658:T1)  [unwired: 2 in, 2 out]
        n344 = Unbundle(w658) -> ("Left"=w634:i32)  [unwired: 1 out]
        n345 = Add(x=w657, y=w658) -> (x+y=w659:T3)
        n346 = Add(x=w634, y=30) -> (x+y=w635:i32)
        n347 = Unbundle(w659) -> ("Width"=w632:u32)  [unwired: 1 out]
        n348 = Greater?(x=w635, y=w645) -> (0:w653:bool)
        n349 = Subtract(x=w632, y=u32 30) -> (x-y=w630:u32)
        n350 = Less?(x=w630, y=w644) -> (x < y?=w652:bool)
        n351 = And(x=w653, y=w652) -> (x .and. y?=w622:bool)
        n352 = property on="disco3" class="Bool (strict)"() -> ("Bounds"=w648:T3)  [unwired: 2 in, 2 out]
        n353 = property on="disco3" class="Bool (strict)"() -> ("Position"=w647:T1)  [unwired: 2 in, 2 out]
        n354 = Unbundle(w647) -> ("Left"=w629:i32)  [unwired: 1 out]
        n355 = Add(x=w648, y=w647) -> (x+y=w646:T3)
        n356 = Add(x=w629, y=30) -> (x+y=w628:i32)
        n357 = Unbundle(w646) -> ("Width"=w626:u32)  [unwired: 1 out]
        n358 = Greater?(x=w628, y=w645) -> (0:w643:bool)
        n359 = Subtract(x=w626, y=u32 30) -> (x-y=w625:u32)
        n360 = Less?(x=w625, y=w644) -> (x < y?=w642:bool)
        n361 = And(x=w643, y=w642) -> (x .and. y?=w623:bool)
        n362 = Compound Arithmetic op=OR(w621, w622, w623) -> (w619:bool)
        n363 = Greater?(x=w609, y=w608) -> (0:w611:cluster{bool, bool})
        n364 = Unbundle(w611) -> (w613:bool, w614:bool)
        n365 = Less?(x=w609, y=w607) -> (x < y?=w612:cluster{bool, bool})
        n366 = And(x=w613, y=w614) -> (x .and. y?=w618:bool)
        n367 = Unbundle(w612) -> (w615:bool, w616:bool)
        n368 = And(x=w615, y=w616) -> (x .and. y?=w617:bool)
        n369 = And(x=w617, y=w618) -> (x .and. y?=w610:bool)
        n370 = Compound Arithmetic op=XOR(w700, w699, w620, w619) -> (w702:bool)
        n371 = case shown="False" w702 {
          tunnel: [FALSE ("Accepted?") TRUE ("Accepted?")] -> w701
          tunnel: w610 -> [w703 _]
          frame False {
            n372 = case shown="True" w703 {
              frame False {
              }
              frame True {
                n373 = local read "# de movimientos"() -> (w707:dbl)
                n374 = Wait (ms)(milliseconds to wait=u32 10) -> ()  [unwired: 1 out]
                n375 = Add(x=w707, y=1.0) -> (x+y=w708:dbl)
                n376 = local write "# de movimientos"(w708) -> ()
              }
            }
          }
          frame True {
            n377 = local read "Position 4"() -> (w710:T1)
            n378 = property on="disco4" class="Bool (strict)"("Position"=w710) -> ()  [unwired: 2 in, 2 out]
          }
        }
        n379 = Exclusive Or(1:w701, 2:w702) -> (0:w660:bool)
      }
      event Mouse Down {
        n380 = event-data() -> ("Coords"=w749:T2)  [unwired: 1 in, 7 out]
        n381 = property on="disco4" class="Bool (strict)"() -> ("Bounds"=w727:T3)  [unwired: 2 in, 2 out]
        n382 = property on="disco4" class="Bool (strict)"() -> ("Position"=w728:T1)  [unwired: 2 in, 2 out]
        "Position 4" <- w728
        n383 = property on="disco1" class="Bool (strict)"() -> ("Bounds"=w738:T3)  [unwired: 2 in, 2 out]
        n384 = property on="disco1" class="Bool (strict)"() -> ("Position"=w737:T1)  [unwired: 2 in, 2 out]
        n385 = Unbundle(w728) -> ("Left"=w717:i32, "Top"=w715:i32)
        n386 = Add(x=w728, y=w727) -> (x+y=w734:T3)
        n387 = Add(x=w737, y=w738) -> (x+y=w735:T3)
        n388 = Unbundle(w737) -> ("Left"=w736:i32, "Top"=w732:i32)
        n389 = Unbundle(w734) -> ("Width"=w716:u32)  [unwired: 1 out]
        n390 = Unbundle(w735) -> ("Width"=w733:u32)  [unwired: 1 out]
        n391 = Greater?(x=w736, y=w717) -> (0:w731:bool)
        n392 = Less?(x=w733, y=w716) -> (x < y?=w730:bool)
        n393 = Less?(x=w732, y=w715) -> (x < y?=w729:bool)
        n394 = Compound Arithmetic op=AND(w731, w730, w729) -> (w711:bool)
        n395 = property on="disco2" class="Bool (strict)"() -> ("Bounds"=w739:T3)  [unwired: 2 in, 2 out]
        n396 = property on="disco2" class="Bool (strict)"() -> ("Position"=w740:T1)  [unwired: 2 in, 2 out]
        n397 = Add(x=w740, y=w739) -> (x+y=w742:T3)
        n398 = Unbundle(w740) -> ("Left"=w741:i32, "Top"=w744:i32)
        n399 = Unbundle(w742) -> ("Width"=w743:u32)  [unwired: 1 out]
        n400 = Greater?(x=w741, y=w717) -> (0:w745:bool)
        n401 = Less?(x=w743, y=w716) -> (x < y?=w746:bool)
        n402 = Less?(x=w744, y=w715) -> (x < y?=w747:bool)
        n403 = Compound Arithmetic op=AND(w745, w746, w747) -> (w712:bool)
        n404 = property on="disco3" class="Bool (strict)"() -> ("Bounds"=w726:T3)  [unwired: 2 in, 2 out]
        n405 = property on="disco3" class="Bool (strict)"() -> ("Position"=w725:T1)  [unwired: 2 in, 2 out]
        n406 = Add(x=w725, y=w726) -> (x+y=w723:T3)
        n407 = Unbundle(w725) -> ("Left"=w724:i32, "Top"=w721:i32)
        n408 = Unbundle(w723) -> ("Width"=w722:u32)  [unwired: 1 out]
        n409 = Greater?(x=w724, y=w717) -> (0:w720:bool)
        n410 = Less?(x=w722, y=w716) -> (x < y?=w719:bool)
        n411 = Less?(x=w721, y=w715) -> (x < y?=w718:bool)
        n412 = Compound Arithmetic op=AND(w720, w719, w718) -> (w713:bool)
        n413 = Compound Arithmetic op=OR(w713, w712, w711) -> (w714:bool)
        n414 = case shown="True" w714 {
          tunnel: w749 -> [w761 _]
          tunnel: [w752 FALSE] -> w748
          tunnel: w728 -> [w751 _]
          tunnel: w727 -> [w750 _]
          frame False {
            n415 = Greater?(x=w761, y=w751) -> (0:w760:cluster{bool, bool})
            n416 = Unbundle(w760) -> (w756:bool, w755:bool)
            n417 = Add(x=w751, y=w750) -> (x+y=w762:T3)
            n418 = And(x=w756, y=w755) -> (x .and. y?=w753:bool)
            n419 = Less?(x=w761, y=w762) -> (x < y?=w759:cluster{bool, bool})
            n420 = Unbundle(w759) -> (w758:bool, w757:bool)
            n421 = And(x=w758, y=w757) -> (x .and. y?=w754:bool)
            n422 = And(x=w753, y=w754) -> (x .and. y?=w752:bool)
          }
          frame True {
          }
        }
      }
    }
    n423 = event shown="[2] \"Pane\": Mouse Up" {
      selector: _ -> [_ _ _ _]
      dyn-events: _ -> [_ _ _ _]
      timeout: _ -> [_ _ _ _]
      tunnel: w13 -> [w336 w337 _ _]
      tunnel: [w336 w337 w375 w424] -> w12
      event Timeout {
        n424 = event-data() -> ()  [unwired: 1 in, 3 out]
      }
      event Mouse Move {
        n425 = event-data() -> ("Coords"=w338:T2)  [unwired: 1 in, 4 out]
        n426 = case shown="True" w337 {
          tunnel: w338 -> [_ w342]
          frame False {
          }
          frame True {
            n427 = property on="disco2" class="Bool (strict)"() -> ("Bounds"=w340:T3)  [unwired: 2 in, 2 out]
            n428 = Divide(x=w340, y=T3 {"Width"=2, "Height"=2}) -> (x/y=w341:cluster{"Width":dbl, "Height":dbl})
            n429 = Subtract(x=w342, y=w341) -> (x-y=w339:cluster{dbl, dbl})
            n430 = property on="disco2" class="Bool (strict)"("Position"=w339) -> ()  [unwired: 2 in, 2 out]
          }
        }
      }
      event Mouse Up {
        n431 = event-data() -> ("Coords"=w346:T2)  [unwired: 1 in, 7 out]
        n432 = property on="medio" class="Bool (strict)"() -> ("Bounds"=w384:T3)  [unwired: 2 in, 2 out]
        n433 = property on="medio" class="Bool (strict)"() -> ("Position"=w385:T1)  [unwired: 2 in, 2 out]
        n434 = property on="disco2" class="Bool (strict)"() -> ("Position"=w345:T1)  [unwired: 2 in, 2 out]
        n435 = property on="disco2" class="Bool (strict)"() -> ("Bounds"=w410:T3)  [unwired: 2 in, 2 out]
        n436 = Add(x=w384, y=w385) -> (x+y=w386:T3)
        n437 = Add(x=w410, y=w345) -> (x+y=w344:T3)
        n438 = Less?(x=w385, y=w344) -> (x < y?=w382:cluster{bool, bool})
        n439 = Greater?(x=w386, y=w345) -> (0:w383:cluster{bool, bool})
        n440 = Unbundle(w382) -> (w378:bool, w379:bool)
        n441 = Unbundle(w383) -> (w376:bool, w377:bool)
        n442 = And(x=w378, y=w379) -> (x .and. y?=w381:bool)
        n443 = And(x=w376, y=w377) -> (x .and. y?=w380:bool)
        n444 = property on="final" class="Bool (strict)"() -> ("Position"=w398:T1)  [unwired: 2 in, 2 out]
        n445 = property on="final" class="Bool (strict)"() -> ("Bounds"=w397:T3)  [unwired: 2 in, 2 out]
        n446 = And(x=w381, y=w380) -> (x .and. y?=w373:bool)
        n447 = Add(x=w397, y=w398) -> (x+y=w387:T3)
        n448 = Add(x=w410, y=w345) -> (x+y=w390:T3)
        n449 = Less?(x=w398, y=w390) -> (x < y?=w389:cluster{bool, bool})
        n450 = Greater?(x=w387, y=w345) -> (0:w388:cluster{bool, bool})
        n451 = Not(x=w373) -> (.not. x?=w412:bool)
        n452 = Unbundle(w389) -> (w394:bool, w393:bool)
        n453 = Unbundle(w388) -> (w396:bool, w395:bool)
        n454 = property on="inicio" class="Bool (strict)"() -> ("Bounds"=w408:T3)  [unwired: 2 in, 2 out]
        n455 = property on="inicio" class="Bool (strict)"() -> ("Position"=w409:T1)  [unwired: 2 in, 2 out]
        n456 = And(x=w394, y=w393) -> (x .and. y?=w391:bool)
        n457 = And(x=w396, y=w395) -> (x .and. y?=w392:bool)
        n458 = And(x=w391, y=w392) -> (x .and. y?=w372:bool)
        n459 = Add(x=w408, y=w409) -> (x+y=w407:T3)
        n460 = Add(x=w410, y=w345) -> (x+y=w367:T3)
        n461 = Less?(x=w409, y=w367) -> (x < y?=w405:cluster{bool, bool})
        n462 = Not(x=w372) -> (.not. x?=w374:bool)
        n463 = Greater?(x=w407, y=w345) -> (0:w406:cluster{bool, bool})
        n464 = Unbundle(w405) -> (w401:bool, w402:bool)
        n465 = Unbundle(w406) -> (w399:bool, w400:bool)
        n466 = property on="disco1" class="Bool (strict)"() -> ("Bounds"=w370:T3)  [unwired: 2 in, 2 out]
        n467 = property on="disco1" class="Bool (strict)"() -> ("Position"=w369:T1)  [unwired: 2 in, 2 out]
        n468 = Unbundle(w345) -> ("Left"=w362:i32)  [unwired: 1 out]
        n469 = And(x=w401, y=w402) -> (x .and. y?=w404:bool)
        n470 = And(x=w399, y=w400) -> (x .and. y?=w403:bool)
        n471 = Unbundle(w369) -> ("Left"=w361:i32)  [unwired: 1 out]
        n472 = Add(x=w370, y=w369) -> (x+y=w368:T3)
        n473 = Add(x=w361, y=30) -> (x+y=w359:i32)
        n474 = And(x=w404, y=w403) -> (x .and. y?=w371:bool)
        n475 = Unbundle(w368) -> ("Width"=w357:u32)  [unwired: 1 out]
        n476 = Greater?(x=w359, y=w362) -> (0:w365:bool)
        n477 = Subtract(x=w357, y=u32 30) -> (x-y=w358:u32)
        n478 = Not(x=w371) -> (.not. x?=w411:bool)
        n479 = Unbundle(w367) -> ("Width"=w366:u32)  [unwired: 1 out]
        n480 = Less?(x=w358, y=w366) -> (x < y?=w364:bool)
        n481 = And(x=w365, y=w364) -> (x .and. y?=w363:bool)
        n482 = Greater?(x=w346, y=w345) -> (0:w348:cluster{bool, bool})
        n483 = Unbundle(w348) -> (w350:bool, w351:bool)
        n484 = Less?(x=w346, y=w344) -> (x < y?=w349:cluster{bool, bool})
        n485 = And(x=w350, y=w351) -> (x .and. y?=w355:bool)
        n486 = Unbundle(w349) -> (w352:bool, w353:bool)
        n487 = Compound Arithmetic op=XOR(w412, w374, w411, w363) -> (w414:bool)
        n488 = And(x=w352, y=w353) -> (x .and. y?=w354:bool)
        n489 = And(x=w354, y=w355) -> (x .and. y?=w347:bool)
        n490 = case shown="False" w414 {
          tunnel: [FALSE ("Accepted?") TRUE ("Accepted?")] -> w413
          tunnel: w347 -> [w415 _]
          frame False {
            n491 = case shown="True" w415 {
              frame False {
              }
              frame True {
                n492 = local read "# de movimientos"() -> (w419:dbl)
                n493 = Wait (ms)(milliseconds to wait=u32 10) -> ()  [unwired: 1 out]
                n494 = Add(x=w419, y=1.0) -> (x+y=w420:dbl)
                n495 = local write "# de movimientos"(w420) -> ()
              }
            }
          }
          frame True {
            n496 = local read "Position 2"() -> (w422:T1)
            n497 = property on="disco2" class="Bool (strict)"("Position"=w422) -> ()  [unwired: 2 in, 2 out]
          }
        }
        n498 = Exclusive Or(1:w413, 2:w414) -> (0:w375:bool)
      }
      event Mouse Down {
        n499 = event-data() -> ("Coords"=w425:T2)  [unwired: 1 in, 7 out]
        n500 = property on="disco2" class="Bool (strict)"() -> ("Bounds"=w427:T3)  [unwired: 2 in, 2 out]
        n501 = property on="disco2" class="Bool (strict)"() -> ("Position"=w426:T1)  [unwired: 2 in, 2 out]
        "Position 2" <- w426
        n502 = property on="disco1" class="Bool (strict)"() -> ("Bounds"=w440:T3)  [unwired: 2 in, 2 out]
        n503 = property on="disco1" class="Bool (strict)"() -> ("Position"=w439:T1)  [unwired: 2 in, 2 out]
        n504 = Unbundle(w426) -> ("Left"=w437:i32, "Top"=w431:i32)
        n505 = Add(x=w426, y=w427) -> (x+y=w435:T3)
        n506 = Add(x=w439, y=w440) -> (x+y=w436:T3)
        n507 = Unbundle(w439) -> ("Left"=w438:i32, "Top"=w432:i32)
        n508 = Unbundle(w435) -> ("Width"=w433:u32)  [unwired: 1 out]
        n509 = Unbundle(w436) -> ("Width"=w434:u32)  [unwired: 1 out]
        n510 = Greater?(x=w438, y=w437) -> (0:w430:bool)
        n511 = Less?(x=w434, y=w433) -> (x < y?=w429:bool)
        n512 = Less?(x=w432, y=w431) -> (x < y?=w428:bool)
        n513 = Compound Arithmetic op=AND(w430, w429, w428) -> (w423:bool)
        n514 = case shown="False" w423 {
          tunnel: w425 -> [w442 _]
          tunnel: [w445 FALSE] -> w424
          tunnel: w427 -> [w444 _]
          tunnel: w426 -> [w443 _]
          tunnel: w425 -> [w441 _]
          frame False {
            n515 = Greater?(x=w441, y=w443) -> (0:w453:cluster{bool, bool})
            n516 = Unbundle(w453) -> (w449:bool, w448:bool)
            n517 = Add(x=w443, y=w444) -> (x+y=w454:T3)
            n518 = And(x=w449, y=w448) -> (x .and. y?=w446:bool)
            n519 = Less?(x=w442, y=w454) -> (x < y?=w452:cluster{bool, bool})
            n520 = Unbundle(w452) -> (w451:bool, w450:bool)
            n521 = And(x=w451, y=w450) -> (x .and. y?=w447:bool)
            n522 = And(x=w446, y=w447) -> (x .and. y?=w445:bool)
          }
          frame True {
          }
        }
      }
    }
    n523 = event shown="[2] \"Pane\": Mouse Up" {
      selector: _ -> [_ _ _ _]
      dyn-events: _ -> [_ _ _ _]
      timeout: _ -> [_ _ _ _]
      tunnel: w11 -> [w250 w251 _ _]
      tunnel: [w250 w251 w273 w325] -> w10
      event Timeout {
        n524 = event-data() -> ()  [unwired: 1 in, 3 out]
      }
      event Mouse Move {
        n525 = event-data() -> ("Coords"=w252:T2)  [unwired: 1 in, 4 out]
        n526 = case shown="False" w251 {
          tunnel: w252 -> [_ w256]
          frame False {
          }
          frame True {
            n527 = property on="disco1" class="Bool (strict)"() -> ("Bounds"=w254:T3)  [unwired: 2 in, 2 out]
            n528 = Divide(x=w254, y=T3 {"Width"=2, "Height"=2}) -> (x/y=w255:cluster{"Width":dbl, "Height":dbl})
            n529 = Subtract(x=w256, y=w255) -> (x-y=w253:cluster{dbl, dbl})
            n530 = property on="disco1" class="Bool (strict)"("Position"=w253) -> ()  [unwired: 2 in, 2 out]
          }
        }
      }
      event Mouse Up {
        n531 = event-data() -> ("Coords"=w260:T2)  [unwired: 1 in, 7 out]
        n532 = property on="medio" class="Bool (strict)"() -> ("Bounds"=w306:T3)  [unwired: 2 in, 2 out]
        n533 = property on="medio" class="Bool (strict)"() -> ("Position"=w305:T1)  [unwired: 2 in, 2 out]
        n534 = property on="disco1" class="Bool (strict)"() -> ("Position"=w261:T1)  [unwired: 2 in, 2 out]
        n535 = property on="disco1" class="Bool (strict)"() -> ("Bounds"=w279:T3)  [unwired: 2 in, 2 out]
        n536 = Add(x=w306, y=w305) -> (x+y=w304:T3)
        n537 = Add(x=w279, y=w261) -> (x+y=w259:T3)
        n538 = Less?(x=w305, y=w259) -> (x < y?=w308:cluster{bool, bool})
        n539 = Greater?(x=w304, y=w261) -> (0:w307:cluster{bool, bool})
        n540 = Unbundle(w308) -> (w312:bool, w311:bool)
        n541 = Unbundle(w307) -> (w314:bool, w313:bool)
        n542 = And(x=w312, y=w311) -> (x .and. y?=w309:bool)
        n543 = And(x=w314, y=w313) -> (x .and. y?=w310:bool)
        n544 = property on="final" class="Bool (strict)"() -> ("Position"=w292:T1)  [unwired: 2 in, 2 out]
        n545 = property on="final" class="Bool (strict)"() -> ("Bounds"=w293:T3)  [unwired: 2 in, 2 out]
        n546 = And(x=w309, y=w310) -> (x .and. y?=w272:bool)
        n547 = Not(x=w272) -> (.not. x?=w276:bool)
        n548 = Add(x=w293, y=w292) -> (x+y=w303:T3)
        n549 = Add(x=w279, y=w261) -> (x+y=w300:T3)
        n550 = Less?(x=w292, y=w300) -> (x < y?=w301:cluster{bool, bool})
        n551 = Greater?(x=w303, y=w261) -> (0:w302:cluster{bool, bool})
        n552 = Unbundle(w301) -> (w296:bool, w297:bool)
        n553 = Unbundle(w302) -> (w294:bool, w295:bool)
        n554 = property on="inicio" class="Bool (strict)"() -> ("Bounds"=w281:T3)  [unwired: 2 in, 2 out]
        n555 = property on="inicio" class="Bool (strict)"() -> ("Position"=w280:T1)  [unwired: 2 in, 2 out]
        n556 = And(x=w296, y=w297) -> (x .and. y?=w299:bool)
        n557 = And(x=w294, y=w295) -> (x .and. y?=w298:bool)
        n558 = And(x=w299, y=w298) -> (x .and. y?=w271:bool)
        n559 = Not(x=w271) -> (.not. x?=w277:bool)
        n560 = Add(x=w281, y=w280) -> (x+y=w282:T3)
        n561 = Add(x=w279, y=w261) -> (x+y=w285:T3)
        n562 = Less?(x=w280, y=w285) -> (x < y?=w284:cluster{bool, bool})
        n563 = Greater?(x=w282, y=w261) -> (0:w283:cluster{bool, bool})
        n564 = Unbundle(w284) -> (w289:bool, w288:bool)
        n565 = Unbundle(w283) -> (w291:bool, w290:bool)
        n566 = Greater?(x=w260, y=w261) -> (0:w269:cluster{bool, bool})
        n567 = And(x=w289, y=w288) -> (x .and. y?=w286:bool)
        n568 = And(x=w291, y=w290) -> (x .and. y?=w287:bool)
        n569 = Unbundle(w269) -> (w267:bool, w266:bool)
        n570 = And(x=w286, y=w287) -> (x .and. y?=w270:bool)
        n571 = Less?(x=w260, y=w259) -> (x < y?=w268:cluster{bool, bool})
        n572 = Not(x=w270) -> (.not. x?=w278:bool)
        n573 = And(x=w267, y=w266) -> (x .and. y?=w262:bool)
        n574 = Unbundle(w268) -> (w265:bool, w264:bool)
        n575 = And(x=w265, y=w264) -> (x .and. y?=w263:bool)
        n576 = And(x=w263, y=w262) -> (x .and. y?=w258:bool)
        n577 = Compound Arithmetic op=XOR(w276, w277, w278) -> (w275:bool)
        n578 = case shown="False" w275 {
          tunnel: [FALSE ("Accepted?") TRUE ("Accepted?")] -> w274
          tunnel: w258 -> [w315 _]
          frame False {
            n579 = case shown="True" w315 {
              frame False {
              }
              frame True {
                n580 = local read "# de movimientos"() -> (w319:dbl)
                n581 = Wait (ms)(milliseconds to wait=u32 10) -> ()  [unwired: 1 out]
                n582 = Add(x=w319, y=1.0) -> (x+y=w320:dbl)
                n583 = local write "# de movimientos"(w320) -> ()
              }
            }
          }
          frame True {
            n584 = local read "Position 1"() -> (w322:T1)
            n585 = property on="disco1" class="Bool (strict)"("Position"=w322) -> ()  [unwired: 2 in, 2 out]
          }
        }
        n586 = Exclusive Or(1:w274, 2:w275) -> (0:w273:bool)
      }
      event Mouse Down {
        n587 = event-data() -> ("Coords"=w334:T2)  [unwired: 1 in, 7 out]
        n588 = property on="disco1" class="Bool (strict)"() -> ("Position"=w323:T1)  [unwired: 2 in, 2 out]
        "Position 1" <- w323
        n589 = property on="disco1" class="Bool (strict)"() -> ("Bounds"=w324:T3)  [unwired: 2 in, 2 out]
        n590 = Greater?(x=w334, y=w323) -> (0:w333:cluster{bool, bool})
        n591 = Unbundle(w333) -> (w329:bool, w328:bool)
        n592 = Add(x=w323, y=w324) -> (x+y=w335:T3)
        n593 = And(x=w329, y=w328) -> (x .and. y?=w326:bool)
        n594 = Less?(x=w334, y=w335) -> (x < y?=w332:cluster{bool, bool})
        n595 = Unbundle(w332) -> (w331:bool, w330:bool)
        n596 = And(x=w331, y=w330) -> (x .and. y?=w327:bool)
        n597 = And(x=w326, y=w327) -> (x .and. y?=w325:bool)
      }
    }
    n598 = case shown="True" "?" {
      frame False {
      }
      frame True {
        w214 = FALSE ("result")
        n599 = property on="solucion de inicio a final 3" class="Str"("Visible"=FALSE) -> ()  [unwired: 2 in, 2 out]
        n600 = case shown="5" "seleccione  # de discos:" {
          frame 0, Default {
          }
          frame 5 {
            n601 = property on="disco3" class="Bool (strict)"("Visible"=TRUE) -> ()  [unwired: 2 in, 2 out]
            n602 = property on="disco4" class="Bool (strict)"("Visible"=TRUE) -> ()  [unwired: 2 in, 2 out]
            n603 = property on="disco2" class="Bool (strict)"("Visible"=TRUE) -> ()  [unwired: 2 in, 2 out]
            n604 = property on="disco1" class="Bool (strict)"("Visible"=TRUE) -> ()  [unwired: 2 in, 2 out]
            n605 = property on="disco5" class="Bool (strict)"("Visible"=TRUE) -> ()  [unwired: 2 in, 2 out]
            n606 = property on="disco4" class="Bool (strict)"("Position"=T1 {"Left"=285, "Top"=429}) -> ()  [unwired: 2 in, 2 out]
            n607 = property on="disco5" class="Bool (strict)"("Position"=T1 {"Left"=271, "Top"=451}) -> ()  [unwired: 2 in, 2 out]
            n608 = property on="disco3" class="Bool (strict)"("Position"=T1 {"Left"=297, "Top"=405}) -> ()  [unwired: 2 in, 2 out]
            n609 = property on="disco2" class="Bool (strict)"("Position"=T1 {"Left"=309, "Top"=381}) -> ()  [unwired: 2 in, 2 out]
            n610 = property on="disco1" class="Bool (strict)"("Position"=T1 {"Left"=321, "Top"=356}) -> ()  [unwired: 2 in, 2 out]
          }
          frame 4 {
            n611 = property on="disco3" class="Bool (strict)"("Visible"=TRUE) -> ()  [unwired: 2 in, 2 out]
            n612 = property on="disco4" class="Bool (strict)"("Visible"=TRUE) -> ()  [unwired: 2 in, 2 out]
            n613 = property on="disco2" class="Bool (strict)"("Visible"=TRUE) -> ()  [unwired: 2 in, 2 out]
            n614 = property on="disco1" class="Bool (strict)"("Visible"=TRUE) -> ()  [unwired: 2 in, 2 out]
            n615 = property on="disco5" class="Bool (strict)"("Visible"=FALSE) -> ()  [unwired: 2 in, 2 out]
            n616 = property on="disco4" class="Bool (strict)"("Position"=T1 {"Left"=285, "Top"=441}) -> ()  [unwired: 2 in, 2 out]
            n617 = property on="disco5" class="Bool (strict)"("Position"=T1 {"Left"=69, "Top"=489}) -> ()  [unwired: 2 in, 2 out]
            n618 = property on="disco3" class="Bool (strict)"("Position"=T1 {"Left"=297, "Top"=417}) -> ()  [unwired: 2 in, 2 out]
            n619 = property on="disco2" class="Bool (strict)"("Position"=T1 {"Left"=309, "Top"=393}) -> ()  [unwired: 2 in, 2 out]
            n620 = property on="disco1" class="Bool (strict)"("Position"=T1 {"Left"=321, "Top"=368}) -> ()  [unwired: 2 in, 2 out]
          }
          frame 3 {
            n621 = property on="disco3" class="Bool (strict)"("Visible"=TRUE) -> ()  [unwired: 2 in, 2 out]
            n622 = property on="disco4" class="Bool (strict)"("Visible"=FALSE) -> ()  [unwired: 2 in, 2 out]
            n623 = property on="disco2" class="Bool (strict)"("Visible"=TRUE) -> ()  [unwired: 2 in, 2 out]
            n624 = property on="disco1" class="Bool (strict)"("Visible"=TRUE) -> ()  [unwired: 2 in, 2 out]
            n625 = property on="disco5" class="Bool (strict)"("Visible"=FALSE) -> ()  [unwired: 2 in, 2 out]
            n626 = property on="disco4" class="Bool (strict)"("Position"=T1 {"Left"=93, "Top"=477}) -> ()  [unwired: 2 in, 2 out]
            n627 = property on="disco5" class="Bool (strict)"("Position"=T1 {"Left"=81, "Top"=501}) -> ()  [unwired: 2 in, 2 out]
            n628 = property on="disco3" class="Bool (strict)"("Position"=T1 {"Left"=297, "Top"=441}) -> ()  [unwired: 2 in, 2 out]
            n629 = property on="disco2" class="Bool (strict)"("Position"=T1 {"Left"=309, "Top"=417}) -> ()  [unwired: 2 in, 2 out]
            n630 = property on="disco1" class="Bool (strict)"("Position"=T1 {"Left"=321, "Top"=392}) -> ()  [unwired: 2 in, 2 out]
          }
        }
        n631 = property on="solucion de inicio a final 4" class="Str"("Visible"=FALSE) -> ()  [unwired: 2 in, 2 out]
        n632 = local write "# de movimientos"(0.0 ("movimientos")) -> ()
        n633 = property on="solucion de inicio a final 5" class="Str"("Visible"=FALSE) -> ()  [unwired: 2 in, 2 out]
        n634 = property class="Str"("Visible"=w214) -> ()  [unwired: 2 in, 2 out]
        n635 = local write "result"(w214) -> ()
      }
    }
    n636 = local write "result"(FALSE ("result")) -> ()
    n637 = local read "seleccione  # de discos:"() -> (w5:u16)
    n638 = case shown="5" w5 {
      frame 0, Default {
      }
      frame 5 {
        n639 = property on="final" class="Bool (strict)"() -> ("Bounds"=w102:T3)  [unwired: 2 in, 2 out]
        n640 = property on="final" class="Bool (strict)"() -> ("Position"=w103:T1)  [unwired: 2 in, 2 out]
        n641 = property on="disco1" class="Bool (strict)"() -> ("Position"=w105:T1)  [unwired: 2 in, 2 out]
        n642 = property on="disco1" class="Bool (strict)"() -> ("Bounds"=w99:T3)  [unwired: 2 in, 2 out]
        n643 = property on="final" class="Bool (strict)"() -> ("Bounds"=w83:T3)  [unwired: 2 in, 2 out]
        n644 = property on="final" class="Bool (strict)"() -> ("Position"=w82:T1)  [unwired: 2 in, 2 out]
        n645 = property on="disco2" class="Bool (strict)"() -> ("Position"=w80:T1)  [unwired: 2 in, 2 out]
        n646 = property on="disco2" class="Bool (strict)"() -> ("Bounds"=w86:T3)  [unwired: 2 in, 2 out]
        n647 = Add(x=w102, y=w103) -> (x+y=w104:T3)
        n648 = Add(x=w83, y=w82) -> (x+y=w81:T3)
        n649 = Add(x=w99, y=w105) -> (x+y=w106:T3)
        n650 = Add(x=w86, y=w80) -> (x+y=w79:T3)
        n651 = Less?(x=w103, y=w106) -> (x < y?=w100:cluster{bool, bool})
        n652 = Less?(x=w82, y=w79) -> (x < y?=w85:cluster{bool, bool})
        n653 = Greater?(x=w104, y=w105) -> (0:w101:cluster{bool, bool})
        n654 = Greater?(x=w81, y=w80) -> (0:w84:cluster{bool, bool})
        n655 = Unbundle(w100) -> (w96:bool, w95:bool)
        n656 = Unbundle(w101) -> (w94:bool, w93:bool)
        n657 = Unbundle(w85) -> (w89:bool, w90:bool)
        n658 = Unbundle(w84) -> (w91:bool, w92:bool)
        n659 = And(x=w96, y=w95) -> (x .and. y?=w98:bool)
        n660 = And(x=w94, y=w93) -> (x .and. y?=w97:bool)
        n661 = And(x=w89, y=w90) -> (x .and. y?=w87:bool)
        n662 = And(x=w91, y=w92) -> (x .and. y?=w88:bool)
        n663 = And(x=w98, y=w97) -> (x .and. y?=w64:bool)
        n664 = And(x=w87, y=w88) -> (x .and. y?=w63:bool)
        n665 = property on="final" class="Bool (strict)"() -> ("Bounds"=w74:T3)  [unwired: 2 in, 2 out]
        n666 = property on="final" class="Bool (strict)"() -> ("Position"=w75:T1)  [unwired: 2 in, 2 out]
        n667 = property on="disco3" class="Bool (strict)"() -> ("Position"=w77:T1)  [unwired: 2 in, 2 out]
        n668 = property on="disco3" class="Bool (strict)"() -> ("Bounds"=w71:T3)  [unwired: 2 in, 2 out]
        n669 = property on="final" class="Bool (strict)"() -> ("Bounds"=w52:T3)  [unwired: 2 in, 2 out]
        n670 = property on="final" class="Bool (strict)"() -> ("Position"=w51:T1)  [unwired: 2 in, 2 out]
        n671 = property on="disco4" class="Bool (strict)"() -> ("Position"=w49:T1)  [unwired: 2 in, 2 out]
        n672 = property on="disco4" class="Bool (strict)"() -> ("Bounds"=w55:T3)  [unwired: 2 in, 2 out]
        n673 = Add(x=w74, y=w75) -> (x+y=w76:T3)
        n674 = Add(x=w71, y=w77) -> (x+y=w78:T3)
        n675 = Add(x=w52, y=w51) -> (x+y=w50:T3)
        n676 = Add(x=w55, y=w49) -> (x+y=w48:T3)
        n677 = Less?(x=w75, y=w78) -> (x < y?=w72:cluster{bool, bool})
        n678 = Less?(x=w51, y=w48) -> (x < y?=w54:cluster{bool, bool})
        n679 = Greater?(x=w76, y=w77) -> (0:w73:cluster{bool, bool})
        n680 = Greater?(x=w50, y=w49) -> (0:w53:cluster{bool, bool})
        n681 = Unbundle(w72) -> (w68:bool, w67:bool)
        n682 = Unbundle(w73) -> (w66:bool, w65:bool)
        n683 = Unbundle(w54) -> (w58:bool, w59:bool)
        n684 = Unbundle(w53) -> (w60:bool, w61:bool)
        n685 = And(x=w68, y=w67) -> (x .and. y?=w70:bool)
        n686 = And(x=w66, y=w65) -> (x .and. y?=w69:bool)
        n687 = And(x=w58, y=w59) -> (x .and. y?=w56:bool)
        n688 = And(x=w60, y=w61) -> (x .and. y?=w57:bool)
        n689 = And(x=w70, y=w69) -> (x .and. y?=w62:bool)
        n690 = And(x=w56, y=w57) -> (x .and. y?=w33:bool)
        n691 = property on="final" class="Bool (strict)"() -> ("Bounds"=w43:T3)  [unwired: 2 in, 2 out]
        n692 = property on="final" class="Bool (strict)"() -> ("Position"=w44:T1)  [unwired: 2 in, 2 out]
        n693 = property on="disco5" class="Bool (strict)"() -> ("Position"=w46:T1)  [unwired: 2 in, 2 out]
        n694 = property on="disco5" class="Bool (strict)"() -> ("Bounds"=w40:T3)  [unwired: 2 in, 2 out]
        n695 = Add(x=w43, y=w44) -> (x+y=w45:T3)
        n696 = Add(x=w40, y=w46) -> (x+y=w47:T3)
        n697 = Less?(x=w44, y=w47) -> (x < y?=w41:cluster{bool, bool})
        n698 = Greater?(x=w45, y=w46) -> (0:w42:cluster{bool, bool})
        n699 = Unbundle(w41) -> (w37:bool, w36:bool)
        n700 = Unbundle(w42) -> (w35:bool, w34:bool)
        n701 = And(x=w37, y=w36) -> (x .and. y?=w39:bool)
        n702 = And(x=w35, y=w34) -> (x .and. y?=w38:bool)
        n703 = And(x=w39, y=w38) -> (x .and. y?=w32:bool)
        n704 = Compound Arithmetic op=AND(w64, w63, w62, w33, w32) -> (w31:bool)
        n705 = local write "result"(w31) -> ()
        n706 = property class="Str"("Visible"=w31) -> ()  [unwired: 2 in, 2 out]
      }
      frame 4 {
        n707 = property on="final" class="Bool (strict)"() -> ("Bounds"=w163:T3)  [unwired: 2 in, 2 out]
        n708 = property on="final" class="Bool (strict)"() -> ("Position"=w164:T1)  [unwired: 2 in, 2 out]
        n709 = property on="disco1" class="Bool (strict)"() -> ("Position"=w166:T1)  [unwired: 2 in, 2 out]
        n710 = property on="disco1" class="Bool (strict)"() -> ("Bounds"=w160:T3)  [unwired: 2 in, 2 out]
        n711 = property on="final" class="Bool (strict)"() -> ("Bounds"=w144:T3)  [unwired: 2 in, 2 out]
        n712 = property on="final" class="Bool (strict)"() -> ("Position"=w143:T1)  [unwired: 2 in, 2 out]
        n713 = property on="disco2" class="Bool (strict)"() -> ("Position"=w141:T1)  [unwired: 2 in, 2 out]
        n714 = property on="disco2" class="Bool (strict)"() -> ("Bounds"=w147:T3)  [unwired: 2 in, 2 out]
        n715 = Add(x=w163, y=w164) -> (x+y=w165:T3)
        n716 = Add(x=w144, y=w143) -> (x+y=w142:T3)
        n717 = Add(x=w160, y=w166) -> (x+y=w167:T3)
        n718 = Add(x=w147, y=w141) -> (x+y=w140:T3)
        n719 = Less?(x=w164, y=w167) -> (x < y?=w161:cluster{bool, bool})
        n720 = Less?(x=w143, y=w140) -> (x < y?=w146:cluster{bool, bool})
        n721 = Greater?(x=w165, y=w166) -> (0:w162:cluster{bool, bool})
        n722 = Greater?(x=w142, y=w141) -> (0:w145:cluster{bool, bool})
        n723 = Unbundle(w161) -> (w157:bool, w156:bool)
        n724 = Unbundle(w162) -> (w155:bool, w154:bool)
        n725 = Unbundle(w146) -> (w150:bool, w151:bool)
        n726 = Unbundle(w145) -> (w152:bool, w153:bool)
        n727 = And(x=w157, y=w156) -> (x .and. y?=w159:bool)
        n728 = And(x=w155, y=w154) -> (x .and. y?=w158:bool)
        n729 = And(x=w150, y=w151) -> (x .and. y?=w148:bool)
        n730 = And(x=w152, y=w153) -> (x .and. y?=w149:bool)
        n731 = And(x=w159, y=w158) -> (x .and. y?=w125:bool)
        n732 = And(x=w148, y=w149) -> (x .and. y?=w124:bool)
        n733 = property on="final" class="Bool (strict)"() -> ("Bounds"=w135:T3)  [unwired: 2 in, 2 out]
        n734 = property on="final" class="Bool (strict)"() -> ("Position"=w136:T1)  [unwired: 2 in, 2 out]
        n735 = property on="disco4" class="Bool (strict)"() -> ("Position"=w138:T1)  [unwired: 2 in, 2 out]
        n736 = property on="disco4" class="Bool (strict)"() -> ("Bounds"=w132:T3)  [unwired: 2 in, 2 out]
        n737 = Add(x=w135, y=w136) -> (x+y=w137:T3)
        n738 = Add(x=w132, y=w138) -> (x+y=w139:T3)
        n739 = Less?(x=w136, y=w139) -> (x < y?=w133:cluster{bool, bool})
        n740 = Greater?(x=w137, y=w138) -> (0:w134:cluster{bool, bool})
        n741 = property on="final" class="Bool (strict)"() -> ("Bounds"=w113:T3)  [unwired: 2 in, 2 out]
        n742 = property on="final" class="Bool (strict)"() -> ("Position"=w112:T1)  [unwired: 2 in, 2 out]
        n743 = property on="disco3" class="Bool (strict)"() -> ("Position"=w110:T1)  [unwired: 2 in, 2 out]
        n744 = property on="disco3" class="Bool (strict)"() -> ("Bounds"=w116:T3)  [unwired: 2 in, 2 out]
        n745 = Unbundle(w133) -> (w129:bool, w128:bool)
        n746 = Unbundle(w134) -> (w127:bool, w126:bool)
        n747 = And(x=w129, y=w128) -> (x .and. y?=w131:bool)
        n748 = And(x=w127, y=w126) -> (x .and. y?=w130:bool)
        n749 = Add(x=w113, y=w112) -> (x+y=w111:T3)
        n750 = Add(x=w116, y=w110) -> (x+y=w109:T3)
        n751 = And(x=w131, y=w130) -> (x .and. y?=w123:bool)
        n752 = Less?(x=w112, y=w109) -> (x < y?=w115:cluster{bool, bool})
        n753 = Greater?(x=w111, y=w110) -> (0:w114:cluster{bool, bool})
        n754 = Unbundle(w115) -> (w119:bool, w120:bool)
        n755 = Unbundle(w114) -> (w121:bool, w122:bool)
        n756 = And(x=w119, y=w120) -> (x .and. y?=w117:bool)
        n757 = And(x=w121, y=w122) -> (x .and. y?=w118:bool)
        n758 = And(x=w117, y=w118) -> (x .and. y?=w108:bool)
        n759 = Compound Arithmetic op=AND(w125, w124, w123, w108) -> (w107:bool)
        n760 = local write "result"(w107) -> ()
        n761 = property class="Str"("Visible"=w107) -> ()  [unwired: 2 in, 2 out]
      }
      frame 3 {
        n762 = property on="final" class="Bool (strict)"() -> ("Bounds"=w209:T3)  [unwired: 2 in, 2 out]
        n763 = property on="final" class="Bool (strict)"() -> ("Position"=w210:T1)  [unwired: 2 in, 2 out]
        n764 = property on="disco1" class="Bool (strict)"() -> ("Position"=w212:T1)  [unwired: 2 in, 2 out]
        n765 = property on="disco1" class="Bool (strict)"() -> ("Bounds"=w206:T3)  [unwired: 2 in, 2 out]
        n766 = property on="final" class="Bool (strict)"() -> ("Bounds"=w190:T3)  [unwired: 2 in, 2 out]
        n767 = property on="final" class="Bool (strict)"() -> ("Position"=w189:T1)  [unwired: 2 in, 2 out]
        n768 = property on="disco2" class="Bool (strict)"() -> ("Position"=w187:T1)  [unwired: 2 in, 2 out]
        n769 = property on="disco2" class="Bool (strict)"() -> ("Bounds"=w193:T3)  [unwired: 2 in, 2 out]
        n770 = Add(x=w209, y=w210) -> (x+y=w211:T3)
        n771 = Add(x=w190, y=w189) -> (x+y=w188:T3)
        n772 = Add(x=w206, y=w212) -> (x+y=w213:T3)
        n773 = Add(x=w193, y=w187) -> (x+y=w186:T3)
        n774 = Less?(x=w210, y=w213) -> (x < y?=w207:cluster{bool, bool})
        n775 = Less?(x=w189, y=w186) -> (x < y?=w192:cluster{bool, bool})
        n776 = Greater?(x=w211, y=w212) -> (0:w208:cluster{bool, bool})
        n777 = Greater?(x=w188, y=w187) -> (0:w191:cluster{bool, bool})
        n778 = Unbundle(w207) -> (w203:bool, w202:bool)
        n779 = Unbundle(w208) -> (w201:bool, w200:bool)
        n780 = Unbundle(w192) -> (w196:bool, w197:bool)
        n781 = Unbundle(w191) -> (w198:bool, w199:bool)
        n782 = And(x=w203, y=w202) -> (x .and. y?=w205:bool)
        n783 = And(x=w201, y=w200) -> (x .and. y?=w204:bool)
        n784 = And(x=w196, y=w197) -> (x .and. y?=w194:bool)
        n785 = And(x=w198, y=w199) -> (x .and. y?=w195:bool)
        n786 = And(x=w205, y=w204) -> (x .and. y?=w171:bool)
        n787 = And(x=w194, y=w195) -> (x .and. y?=w170:bool)
        n788 = property on="final" class="Bool (strict)"() -> ("Bounds"=w181:T3)  [unwired: 2 in, 2 out]
        n789 = property on="final" class="Bool (strict)"() -> ("Position"=w182:T1)  [unwired: 2 in, 2 out]
        n790 = property on="disco3" class="Bool (strict)"() -> ("Position"=w184:T1)  [unwired: 2 in, 2 out]
        n791 = property on="disco3" class="Bool (strict)"() -> ("Bounds"=w178:T3)  [unwired: 2 in, 2 out]
        n792 = Add(x=w181, y=w182) -> (x+y=w183:T3)
        n793 = Add(x=w178, y=w184) -> (x+y=w185:T3)
        n794 = Less?(x=w182, y=w185) -> (x < y?=w179:cluster{bool, bool})
        n795 = Greater?(x=w183, y=w184) -> (0:w180:cluster{bool, bool})
        n796 = Unbundle(w179) -> (w175:bool, w174:bool)
        n797 = Unbundle(w180) -> (w173:bool, w172:bool)
        n798 = And(x=w175, y=w174) -> (x .and. y?=w177:bool)
        n799 = And(x=w173, y=w172) -> (x .and. y?=w176:bool)
        n800 = And(x=w177, y=w176) -> (x .and. y?=w169:bool)
        n801 = Compound Arithmetic op=AND(w171, w170, w169) -> (w168:bool)
        "result" <- w168
        n802 = property class="Str"("Visible"=w168) -> ()  [unwired: 2 in, 2 out]
      }
    }
    n803 = Wait (ms)(milliseconds to wait=u32 10) -> ()  [unwired: 1 out]
    n804 = Wait (ms)(milliseconds to wait=u32 10) -> ()  [unwired: 1 out]
    n805 = case shown="True" "?" {
      frame False {
      }
      frame True {
        n806 = local read "seleccione  # de discos:"() -> (w21:u16)
        n807 = case shown="5" w21 {
          frame 0, Default {
          }
          frame 5 {
            n808 = property on="solucion de inicio a final 5" class="Str"("Visible"=TRUE) -> ()  [unwired: 2 in, 2 out]
            n809 = property on="solucion de inicio a final 3" class="Str"("Visible"=FALSE) -> ()  [unwired: 2 in, 2 out]
            n810 = property on="solucion de inicio a final 4" class="Str"("Visible"=FALSE) -> ()  [unwired: 2 in, 2 out]
          }
          frame 4 {
            n811 = property on="solucion de inicio a final 5" class="Str"("Visible"=FALSE) -> ()  [unwired: 2 in, 2 out]
            n812 = property on="solucion de inicio a final 3" class="Str"("Visible"=FALSE) -> ()  [unwired: 2 in, 2 out]
            n813 = property on="solucion de inicio a final 4" class="Str"("Visible"=TRUE) -> ()  [unwired: 2 in, 2 out]
          }
          frame 3 {
            n814 = property on="solucion de inicio a final 5" class="Str"("Visible"=FALSE) -> ()  [unwired: 2 in, 2 out]
            n815 = property on="solucion de inicio a final 3" class="Str"("Visible"=TRUE) -> ()  [unwired: 2 in, 2 out]
            n816 = property on="solucion de inicio a final 4" class="Str"("Visible"=FALSE) -> ()  [unwired: 2 in, 2 out]
          }
        }
      }
    }
  }
  n817 = property class="Str"("Visible"=FALSE ("result")) -> ()  [unwired: 2 in, 2 out]
  "# de movimientos" <- 0.0 ("movimientos")
